vi "fgv_tim571_databuf.vi"(7 "cmd":T1, 8 "error in":errorcluster, 10 "XYZ_DATA in":cluster{"x":sgl, "y":sgl, "Z":sgl}[](array[cluster])=[{"x"=-0.23617366, "y"=0.44382635, "Z"=2.0646958e-08}, {"x"=-0.2354099, "y"=0.44731313, "Z"=2.0580186e-08}, {"x"=-0.23604421, "y"=0.44938534, "Z"=2.063564e-08}, {"x"=-0.24097842, "y"=0.44728905, "Z"=2.1067002e-08}, {"x"=-0.24088132, "y"=0.4500757, "Z"=2.1058515e-08}, {"x"=-0.2385779, "y"=0.45491207, "Z"=2.0857142e-08}, {"x"=-0.23842053, "y"=0.4576677, "Z"=2.0843386e-08}, {"x"=-0.2360333, "y"=0.46244708, "Z"=2.0634687e-08}, {"x"=-0.23433791, "y"=0.46651757, "Z"=2.0486471e-08}, {"x"=-0.24597977, "y"=0.45851648, "Z"=2.1504235e-08}, {"x"=-0.24352892, "y"=0.46327513, "Z"=2.1289974e-08}, {"x"=-0.24478552, "y"=0.46469545, "Z"=2.139983e-08}, {"x"=-0.24905264, "y"=0.46349877, "Z"=2.1772873e-08}, {"x"=-0.24651532, "y"=0.46820956, "Z"=2.1551054e-08}, {"x"=-0.2507923, "y"=0.46705818, "Z"=2.192496e-08}, {"x"=-0.24513243, "y"=0.47430584, "Z"=2.1430157e-08}, {"x"=-0.24786437, "y"=0.47445863, "Z"=2.1668992e-08}, {"x"=-0.26143128, "y"=0.46576256, "Z"=2.2855048e-08}, {"x"=-0.25101602, "y"=0.4767269, "Z"=2.1944517e-08}, {"x"=-0.26390603, "y"=0.46881858, "Z"=2.3071397e-08}, {"x"=-0.26356125, "y"=0.47159782, "Z"=2.3041256e-08}, {"x"=-0.26476908, "y"=0.47313452, "Z"=2.3146848e-08}, {"x"=-0.0015831427, "y"=0.6787779, "Z"=1.3840273e-10}, {"x"=-0.26715785, "y"=0.47622886, "Z"=2.3355682e-08}, {"x"=-0.27233183, "y"=0.47477728, "Z"=2.3808004e-08}, {"x"=-0.27913585, "y"=0.47218478, "Z"=2.4402832e-08}, {"x"=-0.27631214, "y"=0.4767745, "Z"=2.4155975e-08}, {"x"=-0.2815347, "y"=0.4754463, "Z"=2.4612545e-08}, {"x"=-0.28028262, "y"=0.47883677, "Z"=2.4503084e-08}, {"x"=-0.28144807, "y"=0.4804706, "Z"=2.4604972e-08}, {"x"=-0.28424227, "y"=0.480964, "Z"=2.4849248e-08}, {"x"=-0.29279748, "y"=0.4775015, "Z"=2.5597169e-08}, {"x"=-0.29644778, "y"=0.4775161, "Z"=2.5916288e-08}, {"x"=-0.30922702, "y"=0.4714151, "Z"=2.7033485e-08}, {"x"=-0.31209967, "y"=0.47210872, "Z"=2.7284619e-08}, {"x"=-0.30578443, "y"=0.4788735, "Z"=2.6732524e-08}, {"x"=-0.31701317, "y"=0.4741198, "Z"=2.7714172e-08}, {"x"=-0.31820545, "y"=0.4759674, "Z"=2.7818404e-08}, {"x"=-0.32023188, "y"=0.47728705, "Z"=2.799556e-08}, {"x"=-0.32564586, "y"=0.4765036, "Z"=2.8468866e-08}, {"x"=-0.33533517, "y"=0.47315145, "Z"=2.9315931e-08}, {"x"=-5.450293, "y"=-2.6383529, "Z"=4.7647976e-07}, {"x"=-5.4480753, "y"=-2.593715, "Z"=4.7628586e-07}, {"x"=-5.448104, "y"=-2.550746, "Z"=4.7628836e-07}, {"x"=-5.459038, "y"=-2.5144534, "Z"=4.772442e-07}, {"x"=-5.473198, "y"=-2.4801433, "Z"=4.7848215e-07}, {"x"=-5.4793234, "y"=-2.4413216, "Z"=4.790177e-07}, {"x"=-5.482568, "y"=-2.4010663, "Z"=4.793013e-07}, {"x"=-5.4951506, "y"=-2.3662121, "Z"=4.804013e-07}, {"x"=-5.5013714, "y"=-2.3279579, "Z"=4.809452e-07}, {"x"=-5.519656, "y"=-2.2963793, "Z"=4.8254367e-07}, {"x"=-5.533345, "y"=-2.2623425, "Z"=4.837404e-07}, {"x"=-5.53974, "y"=-2.2245321, "Z"=4.8429945e-07}, {"x"=-5.5441055, "y"=-2.1858287, "Z"=4.846811e-07}, {"x"=-5.5499907, "y"=-2.148081, "Z"=4.851956e-07}, {"x"=-5.5520506, "y"=-2.108567, "Z"=4.8537566e-07}, {"x"=-5.572659, "y"=-2.0784407, "Z"=4.871773e-07}, {"x"=-5.580522, "y"=-2.0420315, "Z"=4.878647e-07}, {"x"=-5.593558, "y"=-2.008223, "Z"=4.890044e-07}, {"x"=-5.610909, "y"=-1.976495, "Z"=4.9052124e-07}, {"x"=-5.6398616, "y"=-1.9501503, "Z"=4.9305237e-07}, {"x"=-5.665971, "y"=-1.9223063, "Z"=4.953349e-07}, {"x"=-5.6819243, "y"=-1.8897145, "Z"=4.967296e-07}, {"x"=-5.683987, "y"=-1.8509235, "Z"=4.9690993e-07}, {"x"=-5.6995296, "y"=-1.8182178, "Z"=4.982687e-07}, {"x"=-5.7130475, "y"=-1.7846243, "Z"=4.994505e-07}, {"x"=-5.740175, "y"=-1.7568197, "Z"=5.01822e-07}, {"x"=-5.7644033, "y"=-1.7276263, "Z"=5.0394016e-07}, {"x"=-5.7727613, "y"=-1.6917732, "Z"=5.046708e-07}, {"x"=-5.77997, "y"=-1.6555295, "Z"=5.0530105e-07}, {"x"=-5.814833, "y"=-1.6303596, "Z"=5.083489e-07}, {"x"=-5.842147, "y"=-1.6019523, "Z"=5.107367e-07}, {"x"=-5.868392, "y"=-1.5729468, "Z"=5.130311e-07}, {"x"=-5.886077, "y"=-1.5405362, "Z"=5.145772e-07}, {"x"=-5.8923306, "y"=-1.5038257, "Z"=5.1512393e-07}, {"x"=-5.9086933, "y"=-1.4708805, "Z"=5.165544e-07}, {"x"=-5.9060388, "y"=-1.4310868, "Z"=5.163223e-07}, {"x"=-5.9021783, "y"=-1.3910661, "Z"=5.159848e-07}, {"x"=-5.8857613, "y"=-1.3469288, "Z"=5.145496e-07}, {"x"=-5.8766103, "y"=-1.305614, "Z"=5.1374957e-07}, {"x"=-5.8567367, "y"=-1.2610137, "Z"=5.120122e-07}, {"x"=-5.8346424, "y"=-1.2160943, "Z"=5.1008067e-07}, {"x"=-5.8446207, "y"=-1.1818175, "Z"=5.10953e-07}, {"x"=-5.8887625, "y"=-1.1582162, "Z"=5.14812e-07}, {"x"=-5.9538646, "y"=-1.1405971, "Z"=5.2050336e-07}, {"x"=-5.9461527, "y"=-1.1004817, "Z"=5.198292e-07}, {"x"=-5.934338, "y"=-1.0593927, "Z"=5.187963e-07}, {"x"=-5.9155188, "y"=-1.0165718, "Z"=5.171511e-07}, {"x"=-5.947433, "y"=-0.98834354, "Z"=5.199411e-07}, {"x"=-6.0419035, "y"=-0.9769929, "Z"=5.2819996e-07}, {"x"=-6.122918, "y"=-0.9609745, "Z"=5.352825e-07}, {"x"=-6.0530334, "y"=-0.90456265, "Z"=5.29173e-07}, {"x"=-5.893567, "y"=-0.8262395, "Z"=5.15232e-07}, {"x"=-5.918724, "y"=-0.7960438, "Z"=5.174313e-07}, {"x"=-5.8494763, "y"=-0.74268264, "Z"=5.1137744e-07}, {"x"=-5.8722486, "y"=-0.7120914, "Z"=5.1336826e-07}, {"x"=-5.9046063, "y"=-0.68353313, "Z"=5.161971e-07}, {"x"=-5.9124384, "y"=-0.6491621, "Z"=5.1688176e-07}, {"x"=-5.9542623, "y"=-0.62222403, "Z"=5.2053815e-07}, {"x"=-5.9969497, "y"=-0.59505194, "Z"=5.2427e-07}, {"x"=-5.9670506, "y"=-0.5524588, "Z"=5.2165615e-07}, {"x"=-5.984905, "y"=-0.51988906, "Z"=5.23217e-07}, {"x"=-6.0271215, "y"=-0.49192494, "Z"=5.269077e-07}, {"x"=-6.070197, "y"=-0.4636951, "Z"=5.306735e-07}, {"x"=-6.0796986, "y"=-0.4289028, "Z"=5.3150416e-07}, {"x"=-6.024004, "y"=-0.3825739, "Z"=5.266352e-07}, {"x"=-5.968964, "y"=-0.33709878, "Z"=5.2182344e-07}, {"x"=-5.966886, "y"=-0.30106133, "Z"=5.2164177e-07}, {"x"=-5.954714, "y"=-0.26351756, "Z"=5.205776e-07}, {"x"=-5.9442844, "y"=-0.22645015, "Z"=5.1966583e-07}, {"x"=-5.9830976, "y"=-0.19678587, "Z"=5.23059e-07}, {"x"=-5.978194, "y"=-0.16057408, "Z"=5.2263033e-07}, {"x"=-5.967126, "y"=-0.123648226, "Z"=5.2166274e-07}, {"x"=-5.9211173, "y"=-0.08240992, "Z"=5.176405e-07}, {"x"=-5.8559747, "y"=-0.039417505, "Z"=5.119456e-07}, {"x"=-5.871979, "y"=-0.0067341924, "Z"=5.1334473e-07}, {"x"=-5.889789, "y"=0.02589035, "Z"=5.149017e-07}, {"x"=-5.8646536, "y"=0.06319648, "Z"=5.127043e-07}, {"x"=-5.8402796, "y"=0.10008913, "Z"=5.1057344e-07}, {"x"=-5.825632, "y"=0.13574708, "Z"=5.0929293e-07}, {"x"=-5.8336806, "y"=0.1692087, "Z"=5.0999654e-07}, {"x"=-5.824593, "y"=0.20412987, "Z"=5.092021e-07}, {"x"=-5.839228, "y"=0.23711291, "Z"=5.104815e-07}, {"x"=-5.8626547, "y"=0.2696217, "Z"=5.1252954e-07}, {"x"=-5.959748, "y"=0.2976503, "Z"=5.210177e-07}, {"x"=-5.9758472, "y"=0.33151048, "Z"=5.224252e-07}, {"x"=-5.952808, "y"=0.367589, "Z"=5.20411e-07}, {"x"=-5.9215603, "y"=0.40376043, "Z"=5.1767927e-07}, {"x"=-5.947047, "y"=0.4372328, "Z"=5.1990736e-07}, {"x"=-5.9403634, "y"=0.47211158, "Z"=5.1932307e-07}, {"x"=-5.9364743, "y"=0.50681686, "Z"=5.189831e-07}, {"x"=-5.9393806, "y"=0.5413065, "Z"=5.192371e-07}, {"x"=-5.9390874, "y"=0.5758766, "Z"=5.192115e-07}, {"x"=-5.930593, "y"=0.61053234, "Z"=5.184689e-07}, {"x"=-5.921897, "y"=0.64508575, "Z"=5.1770866e-07}, {"x"=-5.8849998, "y"=0.6795378, "Z"=5.14483e-07}, {"x"=-5.8789034, "y"=0.7137373, "Z"=5.1395006e-07}, {"x"=-5.881607, "y"=0.74796987, "Z"=5.141864e-07}, {"x"=-5.901109, "y"=0.7825303, "Z"=5.158914e-07}, {"x"=-5.934404, "y"=0.81764466, "Z"=5.1880204e-07}, {"x"=-5.96449, "y"=0.85306275, "Z"=5.214323e-07}, {"x"=-6.003358, "y"=0.88914883, "Z"=5.248302e-07}, {"x"=-6.011032, "y"=0.9244334, "Z"=5.255011e-07}, {"x"=-5.98953, "y"=0.9584675, "Z"=5.2362134e-07}, {"x"=-5.948862, "y"=0.99126697, "Z"=5.2006607e-07}, {"x"=-5.946951, "y"=1.0258671, "Z"=5.1989895e-07}, {"x"=-5.9398484, "y"=1.0601362, "Z"=5.1927805e-07}, {"x"=-5.9375367, "y"=1.0946827, "Z"=5.1907597e-07}, {"x"=-5.9370184, "y"=1.1293662, "Z"=5.190306e-07}, {"x"=-5.924337, "y"=1.1630824, "Z"=5.17922e-07}, {"x"=-5.919434, "y"=1.1973629, "Z"=5.174934e-07}, {"x"=-5.8755016, "y"=1.227981, "Z"=5.1365265e-07}, {"x"=-5.8821654, "y"=1.2631369, "Z"=5.1423524e-07}, {"x"=-5.8836465, "y"=1.2978667, "Z"=5.1436473e-07}, {"x"=-5.877965, "y"=1.3318619, "Z"=5.1386803e-07}, {"x"=-5.872087, "y"=1.3658118, "Z"=5.1335417e-07}, {"x"=-5.8967824, "y"=1.4034905, "Z"=5.155131e-07}, {"x"=-5.9073515, "y"=1.4396942, "Z"=5.1643707e-07}, {"x"=-5.930582, "y"=1.4777781, "Z"=5.1846797e-07}, {"x"=-5.932773, "y"=1.5132372, "Z"=5.186595e-07}, {"x"=-5.9208994, "y"=1.5467211, "Z"=5.1762146e-07}, {"x"=-5.90686, "y"=1.5797939, "Z"=5.163941e-07}, {"x"=-5.9114027, "y"=1.6157031, "Z"=5.1679126e-07}, {"x"=-5.921648, "y"=1.6526682, "Z"=5.176869e-07}, {"x"=-5.952365, "y"=1.6933084, "Z"=5.203723e-07}, {"x"=-5.9562182, "y"=1.7296524, "Z"=5.2070914e-07}, {"x"=-5.960833, "y"=1.7662549, "Z"=5.2111255e-07}, {"x"=-5.955396, "y"=1.8010967, "Z"=5.206373e-07}, {"x"=-5.9360123, "y"=1.8332419, "Z"=5.1894267e-07}, {"x"=-5.9546967, "y"=1.87286, "Z"=5.205761e-07}, {"x"=-5.9525537, "y"=1.9084897, "Z"=5.2038877e-07}, {"x"=-5.962914, "y"=1.9468365, "Z"=5.212945e-07}, {"x"=-5.9730287, "y"=1.9853451, "Z"=5.2217877e-07}, {"x"=-5.9907017, "y"=2.0257678, "Z"=5.2372377e-07}, {"x"=-6.012978, "y"=2.0675642, "Z"=5.256712e-07}, {"x"=-6.018428, "y"=2.1057465, "Z"=5.261477e-07}, {"x"=-5.995456, "y"=2.1371899, "Z"=5.241394e-07}, {"x"=-5.9985223, "y"=2.1749434, "Z"=5.244075e-07}, {"x"=-5.949031, "y"=2.199419, "Z"=5.200808e-07}, {"x"=-5.8984914, "y"=2.2231166, "Z"=5.156625e-07}, {"x"=-5.8836193, "y"=2.2558508, "Z"=5.1436234e-07}, {"x"=-5.9023213, "y"=2.2977157, "Z"=5.159973e-07}, {"x"=-5.9255486, "y"=2.3412008, "Z"=5.180279e-07}, {"x"=-5.926359, "y"=2.3786733, "Z"=5.180988e-07}, {"x"=-5.9173374, "y"=2.4134002, "Z"=5.1731007e-07}, {"x"=-5.9282303, "y"=2.4541004, "Z"=5.1826237e-07}, {"x"=-5.9598885, "y"=2.5014155, "Z"=5.2103e-07}, {"x"=-5.97974, "y"=2.5455847, "Z"=5.227655e-07}, {"x"=-5.9897494, "y"=2.5870125, "Z"=5.2364055e-07}, {"x"=-5.9861636, "y"=2.6242948, "Z"=5.2332706e-07}, {"x"=-6.0307593, "y"=2.6776361, "Z"=5.272257e-07}, {"x"=-6.0275636, "y"=2.715564, "Z"=5.2694634e-07}, {"x"=-6.012784, "y"=2.7496164, "Z"=5.256543e-07}, {"x"=-6.020459, "y"=2.7915087, "Z"=5.2632527e-07}, {"x"=-6.0335007, "y"=2.8355787, "Z"=5.274654e-07}, {"x"=-6.0199194, "y"=2.8702981, "Z"=5.262781e-07}, {"x"=-6.032395, "y"=2.914659, "Z"=5.273687e-07}, {"x"=-6.0249076, "y"=2.9518294, "Z"=5.2671413e-07}, {"x"=-6.0424, "y"=2.9986615, "Z"=5.282434e-07}, {"x"=-6.0418506, "y"=3.0388634, "Z"=5.2819536e-07}, {"x"=-6.0772843, "y"=3.0935318, "Z"=5.312931e-07}, {"x"=-6.1122847, "y"=3.148692, "Z"=5.343529e-07}, {"x"=-6.07932, "y"=3.1766086, "Z"=5.31471e-07}, {"x"=-6.0849957, "y"=3.2204063, "Z"=5.319672e-07}, {"x"=-6.1096983, "y"=3.2725575, "Z"=5.341268e-07}, {"x"=-6.1174703, "y"=3.3179538, "Z"=5.3480625e-07}, {"x"=-6.0983577, "y"=3.3518903, "Z"=5.3313533e-07}, {"x"=-6.0909343, "y"=3.3909798, "Z"=5.324864e-07}, {"x"=-6.100575, "y"=3.4378998, "Z"=5.333292e-07}, {"x"=-6.1198716, "y"=3.489613, "Z"=5.3501617e-07}, {"x"=-6.1170197, "y"=3.5315034, "Z"=5.3476685e-07}, {"x"=-6.096713, "y"=3.5653276, "Z"=5.329916e-07}, {"x"=-6.0960503, "y"=3.6085389, "Z"=5.3293365e-07}, {"x"=-6.0959897, "y"=3.6522777, "Z"=5.3292837e-07}, {"x"=-6.125203, "y"=3.7107499, "Z"=5.354823e-07}, {"x"=-6.119087, "y"=3.7521627, "Z"=5.349476e-07}, {"x"=-6.0886374, "y"=3.781352, "Z"=5.322856e-07}, {"x"=-6.0811543, "y"=3.8222268, "Z"=5.316314e-07}, {"x"=-6.073401, "y"=3.8631191, "Z"=5.3095357e-07}, {"x"=-6.090102, "y"=3.9171696, "Z"=5.3241365e-07}, {"x"=-6.116061, "y"=3.9767406, "Z"=5.3468307e-07}, {"x"=-6.139777, "y"=4.0357633, "Z"=5.367564e-07}, {"x"=-6.2014976, "y"=4.1164994, "Z"=5.421521e-07}, {"x"=-6.416801, "y"=4.2847557, "Z"=5.6097457e-07}, {"x"=-6.5773406, "y"=4.4254436, "Z"=5.750094e-07}, {"x"=-6.599612, "y"=4.489136, "Z"=5.7695644e-07}, {"x"=-6.5730267, "y"=4.524938, "Z"=5.746322e-07}, {"x"=-6.536785, "y"=4.55495, "Z"=5.714639e-07}, {"x"=-6.5372787, "y"=4.6068134, "Z"=5.7150703e-07}, {"x"=-6.4963865, "y"=4.6338573, "Z"=5.6793215e-07}, {"x"=-6.481788, "y"=4.6768293, "Z"=5.666559e-07}, {"x"=-6.3888826, "y"=4.6710234, "Z"=5.585339e-07}, {"x"=-6.3376727, "y"=4.6904745, "Z"=5.5405695e-07}, {"x"=-6.31171, "y"=4.725655, "Z"=5.517872e-07}, {"x"=-6.238583, "y"=4.7301755, "Z"=5.4539424e-07}, {"x"=-6.1814947, "y"=4.744422, "Z"=5.4040345e-07}, {"x"=-6.142764, "y"=4.7703357, "Z"=5.370175e-07}, {"x"=-6.0981383, "y"=4.7920227, "Z"=5.331162e-07}, {"x"=-6.073289, "y"=4.8268633, "Z"=5.309438e-07}, {"x"=-0.0016451083, "y"=0.6811374, "Z"=1.4381994e-10}, {"x"=-6.4596453, "y"=5.2017484, "Z"=5.6472015e-07}, {"x"=-6.502582, "y"=5.288397, "Z"=5.6847375e-07}, {"x"=-6.4837894, "y"=5.331975, "Z"=5.6683086e-07}, {"x"=-6.493028, "y"=5.3960586, "Z"=5.6763855e-07}, {"x"=0.0, "y"=0.68, "Z"=0.0}, {"x"=-7.0161138, "y"=5.9017487, "Z"=6.133682e-07}, {"x"=-6.989613, "y"=5.9454827, "Z"=6.110514e-07}, {"x"=-7.0041914, "y"=6.0206146, "Z"=6.1232583e-07}, {"x"=-6.998339, "y"=6.080819, "Z"=6.1181424e-07}, {"x"=-6.9975395, "y"=6.1454444, "Z"=6.117443e-07}, {"x"=-7.0276036, "y"=6.2350473, "Z"=6.143726e-07}, {"x"=-7.1029325, "y"=6.362039, "Z"=6.209581e-07}, {"x"=-7.2088842, "y"=6.5158896, "Z"=6.3022065e-07}, {"x"=-7.1601167, "y"=6.5456853, "Z"=6.259573e-07}, {"x"=-7.1512794, "y"=6.6082983, "Z"=6.251847e-07}, {"x"=-7.1205034, "y"=6.653012, "Z"=6.2249416e-07}, {"x"=-7.086399, "y"=6.6949787, "Z"=6.1951266e-07}, {"x"=-7.048255, "y"=6.7334933, "Z"=6.16178e-07}, {"x"=-7.0808544, "y"=6.833427, "Z"=6.1902796e-07}, {"x"=-7.048694, "y"=6.877815, "Z"=6.162164e-07}, {"x"=-7.003556, "y"=6.910737, "Z"=6.122703e-07}, {"x"=-7.0861115, "y"=7.058415, "Z"=6.1948754e-07}, {"x"=-7.1871443, "y"=7.225441, "Z"=6.283201e-07}, {"x"=-7.2004256, "y"=7.3145723, "Z"=6.294812e-07}, {"x"=-7.218032, "y"=7.408851, "Z"=6.310204e-07}, {"x"=-7.145303, "y"=7.4191637, "Z"=6.246622e-07}, {"x"=-7.019162, "y"=7.377773, "Z"=6.1363465e-07}, {"x"=-6.992312, "y"=7.4302983, "Z"=6.112873e-07}, {"x"=-6.945772, "y"=7.4638724, "Z"=6.072187e-07}, {"x"=-6.8535547, "y"=7.45215, "Z"=5.991568e-07}, {"x"=-6.8373823, "y"=7.5152345, "Z"=5.9774294e-07}, {"x"=-6.828441, "y"=7.586181, "Z"=5.969613e-07}, {"x"=-6.711966, "y"=7.547832, "Z"=5.867787e-07}, {"x"=-6.6600904, "y"=7.5745335, "Z"=5.822436e-07}, {"x"=-6.76213, "y"=7.762151, "Z"=5.9116417e-07}, {"x"=-6.7496448, "y"=7.8319125, "Z"=5.9007266e-07}, {"x"=0.0, "y"=0.68, "Z"=0.0}, {"x"=0.0, "y"=0.68, "Z"=0.0}, {"x"=0.0, "y"=0.68, "Z"=0.0}, {"x"=0.0, "y"=0.68, "Z"=0.0}, {"x"=0.0, "y"=0.68, "Z"=0.0}, {"x"=0.0, "y"=0.68, "Z"=0.0}, {"x"=0.0, "y"=0.68, "Z"=0.0}, {"x"=0.0, "y"=0.68, "Z"=0.0}, {"x"=0.0, "y"=0.68, "Z"=0.0}, {"x"=0.0, "y"=0.68, "Z"=0.0}, {"x"=-6.6047463, "y"=8.642182, "Z"=5.774053e-07}, {"x"=-6.5773363, "y"=8.70367, "Z"=5.75009e-07}, {"x"=-6.549433, "y"=8.765107, "Z"=5.7256966e-07}, {"x"=0.0, "y"=0.68, "Z"=0.0}, {"x"=0.0, "y"=0.68, "Z"=0.0}, {"x"=0.0, "y"=0.68, "Z"=0.0}, {"x"=0.0, "y"=0.68, "Z"=0.0}, {"x"=0.0, "y"=0.68, "Z"=0.0}, {"x"=0.0, "y"=0.68, "Z"=0.0}, {"x"=0.0, "y"=0.68, "Z"=0.0}, {"x"=0.0, "y"=0.68, "Z"=0.0}, {"x"=0.0, "y"=0.68, "Z"=0.0}, {"x"=0.0, "y"=0.68, "Z"=0.0}, {"x"=0.0, "y"=0.68, "Z"=0.0}, {"x"=0.0, "y"=0.68, "Z"=0.0}, {"x"=0.0, "y"=0.68, "Z"=0.0}, {"x"=-6.206232, "y"=9.763209, "Z"=5.4256606e-07}, {"x"=0.0, "y"=0.68, "Z"=0.0}, {"x"=0.0, "y"=0.68, "Z"=0.0}, {"x"=0.0, "y"=0.68, "Z"=0.0}, {"x"=0.0, "y"=0.68, "Z"=0.0}, {"x"=0.0, "y"=0.68, "Z"=0.0}, {"x"=0.0, "y"=0.68, "Z"=0.0}, {"x"=0.0, "y"=0.68, "Z"=0.0}, {"x"=0.0, "y"=0.68, "Z"=0.0}, {"x"=0.0, "y"=0.68, "Z"=0.0}, {"x"=0.0, "y"=0.68, "Z"=0.0}, {"x"=0.0, "y"=0.68, "Z"=0.0}, {"x"=0.0, "y"=0.68, "Z"=0.0}, {"x"=0.0, "y"=0.68, "Z"=0.0}, {"x"=0.0, "y"=0.68, "Z"=0.0}, {"x"=0.0, "y"=0.68, "Z"=0.0}, {"x"=0.0, "y"=0.68, "Z"=0.0}, {"x"=0.0, "y"=0.68, "Z"=0.0}, {"x"=0.0, "y"=0.68, "Z"=0.0}, {"x"=0.0, "y"=0.68, "Z"=0.0}, {"x"=0.0, "y"=0.68, "Z"=0.0}, {"x"=0.0, "y"=0.68, "Z"=0.0}, {"x"=0.0, "y"=0.68, "Z"=0.0}, {"x"=0.0, "y"=0.68, "Z"=0.0}, {"x"=0.0, "y"=0.68, "Z"=0.0}, {"x"=0.0, "y"=0.68, "Z"=0.0}, {"x"=0.0, "y"=0.68, "Z"=0.0}, {"x"=0.0, "y"=0.68, "Z"=0.0}, {"x"=0.0, "y"=0.68, "Z"=0.0}, {"x"=0.0, "y"=0.68, "Z"=0.0}, {"x"=0.0, "y"=0.68, "Z"=0.0}, {"x"=0.0, "y"=0.68, "Z"=0.0}, {"x"=0.0, "y"=0.68, "Z"=0.0}, {"x"=0.0, "y"=0.68, "Z"=0.0}, {"x"=0.0, "y"=0.68, "Z"=0.0}, {"x"=0.0, "y"=0.68, "Z"=0.0}, {"x"=0.0, "y"=0.68, "Z"=0.0}, {"x"=0.0, "y"=0.68, "Z"=0.0}, {"x"=0.0, "y"=0.68, "Z"=0.0}, {"x"=0.0, "y"=0.68, "Z"=0.0}, {"x"=0.0, "y"=0.68, "Z"=0.0}, {"x"=0.0, "y"=0.68, "Z"=0.0}, {"x"=0.0, "y"=0.68, "Z"=0.0}, {"x"=0.0, "y"=0.68, "Z"=0.0}, {"x"=0.0, "y"=0.68, "Z"=0.0}, {"x"=0.0, "y"=0.68, "Z"=0.0}, {"x"=0.0, "y"=0.68, "Z"=0.0}, {"x"=0.0, "y"=0.68, "Z"=0.0}, {"x"=0.0, "y"=0.68, "Z"=0.0}, {"x"=0.0, "y"=0.68, "Z"=0.0}, {"x"=0.0, "y"=0.68, "Z"=0.0}, {"x"=0.0, "y"=0.68, "Z"=0.0}, {"x"=0.0, "y"=0.68, "Z"=0.0}, {"x"=0.0, "y"=0.68, "Z"=0.0}, {"x"=0.0, "y"=0.68, "Z"=0.0}, {"x"=0.0, "y"=0.68, "Z"=0.0}, {"x"=0.0, "y"=0.68, "Z"=0.0}, {"x"=0.0, "y"=0.68, "Z"=0.0}, {"x"=0.0, "y"=0.68, "Z"=0.0}, {"x"=0.0, "y"=0.68, "Z"=0.0}, {"x"=0.0, "y"=0.68, "Z"=0.0}, {"x"=0.0, "y"=0.68, "Z"=0.0}, {"x"=0.0, "y"=0.68, "Z"=0.0}, {"x"=0.0, "y"=0.68, "Z"=0.0}, {"x"=0.0, "y"=0.68, "Z"=0.0}, {"x"=0.0, "y"=0.68, "Z"=0.0}, {"x"=0.0, "y"=0.68, "Z"=0.0}, {"x"=0.0, "y"=0.68, "Z"=0.0}, {"x"=0.0, "y"=0.68, "Z"=0.0}, {"x"=0.0, "y"=0.68, "Z"=0.0}, {"x"=0.0, "y"=0.68, "Z"=0.0}, {"x"=0.0, "y"=0.68, "Z"=0.0}, {"x"=0.0, "y"=0.68, "Z"=0.0}, {"x"=0.0, "y"=0.68, "Z"=0.0}, {"x"=0.0, "y"=0.68, "Z"=0.0}, {"x"=0.0, "y"=0.68, "Z"=0.0}, {"x"=0.0, "y"=0.68, "Z"=0.0}, {"x"=0.0, "y"=0.68, "Z"=0.0}, {"x"=0.0, "y"=0.68, "Z"=0.0}, {"x"=0.0, "y"=0.68, "Z"=0.0}, {"x"=0.0, "y"=0.68, "Z"=0.0}, {"x"=0.0, "y"=0.68, "Z"=0.0}, {"x"=0.0, "y"=0.68, "Z"=0.0}, {"x"=0.0, "y"=0.68, "Z"=0.0}, {"x"=0.0, "y"=0.68, "Z"=0.0}, {"x"=0.0, "y"=0.68, "Z"=0.0}, {"x"=0.0, "y"=0.68, "Z"=0.0}, {"x"=0.0, "y"=0.68, "Z"=0.0}, {"x"=0.0, "y"=0.68, "Z"=0.0}, {"x"=0.0, "y"=0.68, "Z"=0.0}, {"x"=0.0, "y"=0.68, "Z"=0.0}, {"x"=0.0, "y"=0.68, "Z"=0.0}, {"x"=0.0, "y"=0.68, "Z"=0.0}, {"x"=0.0, "y"=0.68, "Z"=0.0}, {"x"=0.0, "y"=0.68, "Z"=0.0}, {"x"=0.0, "y"=0.68, "Z"=0.0}, {"x"=0.0, "y"=0.68, "Z"=0.0}, {"x"=0.0, "y"=0.68, "Z"=0.0}, {"x"=0.0, "y"=0.68, "Z"=0.0}, {"x"=0.0, "y"=0.68, "Z"=0.0}, {"x"=0.0, "y"=0.68, "Z"=0.0}, {"x"=0.0, "y"=0.68, "Z"=0.0}, {"x"=0.0, "y"=0.68, "Z"=0.0}, {"x"=0.0, "y"=0.68, "Z"=0.0}, {"x"=0.0, "y"=0.68, "Z"=0.0}, {"x"=0.0, "y"=0.68, "Z"=0.0}, {"x"=0.0, "y"=0.68, "Z"=0.0}, {"x"=0.0, "y"=0.68, "Z"=0.0}, {"x"=0.0, "y"=0.68, "Z"=0.0}, {"x"=0.0, "y"=0.68, "Z"=0.0}, {"x"=0.0, "y"=0.68, "Z"=0.0}, {"x"=0.0, "y"=0.68, "Z"=0.0}, {"x"=0.0, "y"=0.68, "Z"=0.0}, {"x"=0.0, "y"=0.68, "Z"=0.0}, {"x"=0.0, "y"=0.68, "Z"=0.0}, {"x"=0.0, "y"=0.68, "Z"=0.0}, {"x"=0.0, "y"=0.68, "Z"=0.0}, {"x"=0.0, "y"=0.68, "Z"=0.0}, {"x"=0.0, "y"=0.68, "Z"=0.0}, {"x"=0.0, "y"=0.68, "Z"=0.0}, {"x"=0.0, "y"=0.68, "Z"=0.0}, {"x"=0.0, "y"=0.68, "Z"=0.0}, {"x"=0.0, "y"=0.68, "Z"=0.0}, {"x"=0.0, "y"=0.68, "Z"=0.0}, {"x"=0.0, "y"=0.68, "Z"=0.0}, {"x"=0.0, "y"=0.68, "Z"=0.0}, {"x"=0.0, "y"=0.68, "Z"=0.0}, {"x"=0.0, "y"=0.68, "Z"=0.0}, {"x"=0.0, "y"=0.68, "Z"=0.0}, {"x"=0.0, "y"=0.68, "Z"=0.0}, {"x"=0.0, "y"=0.68, "Z"=0.0}, {"x"=0.0, "y"=0.68, "Z"=0.0}, {"x"=0.0, "y"=0.68, "Z"=0.0}, {"x"=0.0, "y"=0.68, "Z"=0.0}, {"x"=0.0, "y"=0.68, "Z"=0.0}, {"x"=0.0, "y"=0.68, "Z"=0.0}, {"x"=0.0, "y"=0.68, "Z"=0.0}, {"x"=0.0, "y"=0.68, "Z"=0.0}, {"x"=0.0, "y"=0.68, "Z"=0.0}, {"x"=0.0, "y"=0.68, "Z"=0.0}, {"x"=0.0, "y"=0.68, "Z"=0.0}, {"x"=0.0, "y"=0.68, "Z"=0.0}, {"x"=0.0, "y"=0.68, "Z"=0.0}, {"x"=0.0, "y"=0.68, "Z"=0.0}, {"x"=0.0, "y"=0.68, "Z"=0.0}, {"x"=0.0, "y"=0.68, "Z"=0.0}, {"x"=0.0, "y"=0.68, "Z"=0.0}, {"x"=0.0, "y"=0.68, "Z"=0.0}, {"x"=0.0, "y"=0.68, "Z"=0.0}, {"x"=0.0, "y"=0.68, "Z"=0.0}, {"x"=0.0, "y"=0.68, "Z"=0.0}, {"x"=0.0, "y"=0.68, "Z"=0.0}, {"x"=0.0, "y"=0.68, "Z"=0.0}, {"x"=0.0, "y"=0.68, "Z"=0.0}, {"x"=0.0, "y"=0.68, "Z"=0.0}, {"x"=0.0, "y"=0.68, "Z"=0.0}, {"x"=0.0, "y"=0.68, "Z"=0.0}, {"x"=0.0, "y"=0.68, "Z"=0.0}, {"x"=0.0, "y"=0.68, "Z"=0.0}, {"x"=0.0, "y"=0.68, "Z"=0.0}, {"x"=0.0, "y"=0.68, "Z"=0.0}, {"x"=0.0, "y"=0.68, "Z"=0.0}, {"x"=0.0, "y"=0.68, "Z"=0.0}, {"x"=0.0, "y"=0.68, "Z"=0.0}, {"x"=0.0, "y"=0.68, "Z"=0.0}, {"x"=0.0, "y"=0.68, "Z"=0.0}, {"x"=0.0, "y"=0.68, "Z"=0.0}, {"x"=0.0, "y"=0.68, "Z"=0.0}, {"x"=0.0, "y"=0.68, "Z"=0.0}, {"x"=0.0, "y"=0.68, "Z"=0.0}, {"x"=0.0, "y"=0.68, "Z"=0.0}, {"x"=0.0, "y"=0.68, "Z"=0.0}, {"x"=0.0, "y"=0.68, "Z"=0.0}, {"x"=0.0, "y"=0.68, "Z"=0.0}, {"x"=0.0, "y"=0.68, "Z"=0.0}, {"x"=0.0, "y"=0.68, "Z"=0.0}, {"x"=0.0, "y"=0.68, "Z"=0.0}, {"x"=0.0, "y"=0.68, "Z"=0.0}, {"x"=0.0, "y"=0.68, "Z"=0.0}, {"x"=0.0, "y"=0.68, "Z"=0.0}, {"x"=0.0, "y"=0.68, "Z"=0.0}, {"x"=0.0, "y"=0.68, "Z"=0.0}, {"x"=0.0, "y"=0.68, "Z"=0.0}, {"x"=0.0, "y"=0.68, "Z"=0.0}, {"x"=0.0, "y"=0.68, "Z"=0.0}, {"x"=0.0, "y"=0.68, "Z"=0.0}, {"x"=0.0, "y"=0.68, "Z"=0.0}, {"x"=0.0, "y"=0.68, "Z"=0.0}, {"x"=0.0, "y"=0.68, "Z"=0.0}, {"x"=0.0, "y"=0.68, "Z"=0.0}, {"x"=0.0, "y"=0.68, "Z"=0.0}, {"x"=0.0, "y"=0.68, "Z"=0.0}, {"x"=0.0, "y"=0.68, "Z"=0.0}, {"x"=0.0, "y"=0.68, "Z"=0.0}, {"x"=0.0, "y"=0.68, "Z"=0.0}, {"x"=0.0, "y"=0.68, "Z"=0.0}, {"x"=0.0, "y"=0.68, "Z"=0.0}, {"x"=0.0, "y"=0.68, "Z"=0.0}, {"x"=5.316029, "y"=9.30421, "Z"=-4.6474202e-07}, {"x"=5.351277, "y"=9.249391, "Z"=-4.6782347e-07}, {"x"=5.3833942, "y"=9.1902275, "Z"=-4.7063128e-07}, {"x"=0.0, "y"=0.68, "Z"=0.0}, {"x"=0.0, "y"=0.68, "Z"=0.0}, {"x"=0.0, "y"=0.68, "Z"=0.0}, {"x"=5.9229383, "y"=9.5779505, "Z"=-5.177997e-07}, {"x"=6.0003104, "y"=9.581489, "Z"=-5.245638e-07}, {"x"=6.0999103, "y"=9.616638, "Z"=-5.332711e-07}, {"x"=6.13701, "y"=9.559614, "Z"=-5.3651445e-07}, {"x"=6.04924, "y"=9.324669, "Z"=-5.288414e-07}, {"x"=5.994213, "y"=9.140826, "Z"=-5.240307e-07}, {"x"=6.1913676, "y"=9.312213, "Z"=-5.4126656e-07}, {"x"=6.417741, "y"=9.518808, "Z"=-5.610567e-07}, {"x"=6.4666796, "y"=9.478103, "Z"=-5.653351e-07}, {"x"=0.0, "y"=0.68, "Z"=0.0}, {"x"=5.907469, "y"=8.524375, "Z"=-5.164473e-07}, {"x"=5.778412, "y"=8.26083, "Z"=-5.051648e-07}, {"x"=5.659322, "y"=8.015687, "Z"=-4.9475364e-07}, {"x"=5.704976, "y"=7.9865823, "Z"=-4.9874484e-07}, {"x"=5.8186827, "y"=8.043502, "Z"=-5.086854e-07}, {"x"=5.830191, "y"=7.9704795, "Z"=-5.096915e-07}, {"x"=5.8221755, "y"=7.874254, "Z"=-5.0899075e-07}, {"x"=5.875332, "y"=7.85419, "Z"=-5.136378e-07}, {"x"=5.902928, "y"=7.802952, "Z"=-5.1605036e-07}, {"x"=6.019442, "y"=7.858143, "Z"=-5.2623636e-07}, {"x"=6.089565, "y"=7.856555, "Z"=-5.3236664e-07}, {"x"=6.180717, "y"=7.878672, "Z"=-5.4033546e-07}, {"x"=6.277578, "y"=7.9060087, "Z"=-5.488033e-07}, {"x"=6.357798, "y"=7.9129314, "Z"=-5.5581637e-07}, {"x"=6.4901466, "y"=7.977448, "Z"=-5.673866e-07}, {"x"=6.529143, "y"=7.935854, "Z"=-5.707958e-07}, {"x"=6.6789546, "y"=8.016062, "Z"=-5.8389276e-07}, {"x"=6.8692126, "y"=8.137428, "Z"=-6.0052565e-07}, {"x"=7.0672393, "y"=8.263409, "Z"=-6.1783766e-07}, {"x"=7.177091, "y"=8.292017, "Z"=-6.2744124e-07}, {"x"=0.0, "y"=0.68, "Z"=0.0}, {"x"=7.342941, "y"=8.288593, "Z"=-6.419403e-07}, {"x"=7.3556395, "y"=8.213552, "Z"=-6.4305044e-07}, {"x"=7.387392, "y"=8.158542, "Z"=-6.4582633e-07}, {"x"=7.4032025, "y"=8.087855, "Z"=-6.4720854e-07}, {"x"=7.436927, "y"=8.035523, "Z"=-6.501568e-07}, {"x"=0.0, "y"=0.68, "Z"=0.0}, {"x"=0.0, "y"=0.68, "Z"=0.0}, {"x"=0.0, "y"=0.68, "Z"=0.0}, {"x"=0.0, "y"=0.68, "Z"=0.0}, {"x"=6.662852, "y"=6.8971677, "Z"=-5.8248503e-07}, {"x"=6.7562423, "y"=6.911185, "Z"=-5.9064945e-07}, {"x"=0.0014780493, "y"=0.68134737, "Z"=-1.2921518e-10}, {"x"=6.9263463, "y"=6.920517, "Z"=-6.055204e-07}, {"x"=7.0080867, "y"=6.920687, "Z"=-6.126664e-07}, {"x"=5.7576256, "y"=5.74741, "Z"=-5.033476e-07}, {"x"=5.7296643, "y"=5.6639524, "Z"=-5.009032e-07}, {"x"=6.963505, "y"=6.666409, "Z"=-6.087689e-07}, {"x"=6.947913, "y"=6.583066, "Z"=-6.0740587e-07}, {"x"=6.831265, "y"=6.415871, "Z"=-5.9720816e-07}, {"x"=6.7529287, "y"=6.2834435, "Z"=-5.903598e-07}, {"x"=6.694938, "y"=6.169878, "Z"=-5.852901e-07}, {"x"=6.7267604, "y"=6.13084, "Z"=-5.8807206e-07}, {"x"=6.7380595, "y"=6.075366, "Z"=-5.890599e-07}, {"x"=6.7583523, "y"=6.0273914, "Z"=-5.908339e-07}, {"x"=6.7743764, "y"=5.976284, "Z"=-5.922348e-07}, {"x"=6.805071, "y"=5.936787, "Z"=-5.9491816e-07}, {"x"=6.807713, "y"=5.875877, "Z"=-5.951492e-07}, {"x"=6.834629, "y"=5.8337793, "Z"=-5.9750226e-07}, {"x"=6.8364263, "y"=5.773024, "Z"=-5.976594e-07}, {"x"=6.8280845, "y"=5.7053103, "Z"=-5.969301e-07}, {"x"=6.8183784, "y"=5.637279, "Z"=-5.960816e-07}, {"x"=6.824358, "y"=5.581198, "Z"=-5.966043e-07}, {"x"=6.8486753, "y"=5.5385237, "Z"=-5.987302e-07}, {"x"=6.840788, "y"=5.4733524, "Z"=-5.980407e-07}, {"x"=6.846354, "y"=5.4181128, "Z"=-5.9852727e-07}, {"x"=6.83087, "y"=5.3488636, "Z"=-5.9717365e-07}, {"x"=6.8380218, "y"=5.295621, "Z"=-5.977989e-07}, {"x"=6.8081737, "y"=5.2180495, "Z"=-5.951894e-07}, {"x"=6.834457, "y"=5.178369, "Z"=-5.974872e-07}, {"x"=5.3789005, "y"=4.175662, "Z"=-4.7023843e-07}, {"x"=5.3940945, "y"=4.1410728, "Z"=-4.7156672e-07}, {"x"=5.5298705, "y"=4.1829486, "Z"=-4.834366e-07}, {"x"=6.9839015, "y"=5.0472975, "Z"=-6.1055204e-07}, {"x"=6.9955735, "y"=4.9981933, "Z"=-6.115725e-07}, {"x"=7.009473, "y"=4.9506617, "Z"=-6.127876e-07}, {"x"=5.7307115, "y"=4.126, "Z"=-5.009947e-07}, {"x"=5.9260955, "y"=4.1967134, "Z"=-5.180757e-07}, {"x"=0.0, "y"=0.68, "Z"=0.0}, {"x"=6.677475, "y"=4.538273, "Z"=-5.837634e-07}, {"x"=6.6329126, "y"=4.4612293, "Z"=-5.798676e-07}, {"x"=6.657411, "y"=4.4240513, "Z"=-5.8200936e-07}, {"x"=6.6204896, "y"=4.3527584, "Z"=-5.7878157e-07}, {"x"=6.6075296, "y"=4.2954636, "Z"=-5.7764856e-07}, {"x"=6.6134887, "y"=4.248892, "Z"=-5.7816953e-07}, {"x"=6.591764, "y"=4.187811, "Z"=-5.762703e-07}, {"x"=6.5704393, "y"=4.1275682, "Z"=-5.7440604e-07}, {"x"=6.549526, "y"=4.068153, "Z"=-5.725778e-07}, {"x"=6.5477443, "y"=4.019093, "Z"=-5.72422e-07}, {"x"=6.53936, "y"=3.967025, "Z"=-5.71689e-07}, {"x"=6.5494094, "y"=3.92449, "Z"=-5.7256756e-07}, {"x"=6.5501995, "y"=3.8775625, "Z"=-5.726366e-07}, {"x"=6.565085, "y"=3.8376713, "Z"=-5.7393794e-07}, {"x"=6.5896683, "y"=3.8024251, "Z"=-5.760871e-07}, {"x"=6.591409, "y"=3.7564263, "Z"=-5.762393e-07}, {"x"=6.62464, "y"=3.7251313, "Z"=-5.791444e-07}, {"x"=6.638598, "y"=3.6848936, "Z"=-5.8036466e-07}, {"x"=6.6258235, "y"=3.6327922, "Z"=-5.792479e-07}, {"x"=6.641972, "y"=3.5937972, "Z"=-5.806596e-07}, {"x"=6.623005, "y"=3.539651, "Z"=-5.790015e-07}, {"x"=6.653333, "y"=3.5069413, "Z"=-5.8165284e-07}, {"x"=6.695499, "y"=3.4789894, "Z"=-5.853391e-07}, {"x"=6.711668, "y"=3.4399934, "Z"=-5.8675266e-07}, {"x"=6.7081413, "y"=3.3930302, "Z"=-5.8644434e-07}, {"x"=6.731244, "y"=3.3569183, "Z"=-5.8846405e-07}, {"x"=6.760672, "y"=3.3231783, "Z"=-5.910367e-07}, {"x"=6.7778006, "y"=3.2845232, "Z"=-5.9253415e-07}, {"x"=6.7741265, "y"=3.2379863, "Z"=-5.922129e-07}, {"x"=6.7776413, "y"=3.194363, "Z"=-5.925202e-07}, {"x"=6.7780595, "y"=3.1497586, "Z"=-5.925568e-07}, {"x"=6.8214993, "y"=3.1207314, "Z"=-5.963544e-07}, {"x"=6.8157687, "y"=3.074049, "Z"=-5.958534e-07}, {"x"=6.8295803, "y"=3.0343602, "Z"=-5.970609e-07}, {"x"=6.8545275, "y"=2.9984365, "Z"=-5.9924184e-07}, {"x"=6.8821354, "y"=2.9632466, "Z"=-6.0165536e-07}, {"x"=6.8658214, "y"=2.9135835, "Z"=-6.0022916e-07}, {"x"=6.869171, "y"=2.8705678, "Z"=-6.00522e-07}, {"x"=6.8951607, "y"=2.8347478, "Z"=-6.027941e-07}, {"x"=6.913316, "y"=2.7963574, "Z"=-6.043813e-07}, {"x"=6.890068, "y"=2.7454813, "Z"=-6.023489e-07}, {"x"=6.8664637, "y"=2.6949475, "Z"=-6.002853e-07}, {"x"=6.8723016, "y"=2.653314, "Z"=-6.0079566e-07}, {"x"=6.8682604, "y"=2.6089773, "Z"=-6.004424e-07}, {"x"=6.8909373, "y"=2.5721684, "Z"=-6.0242485e-07}, {"x"=6.876716, "y"=2.5253122, "Z"=-6.011816e-07}, {"x"=6.8844323, "y"=2.4845173, "Z"=-6.018562e-07}, {"x"=6.893844, "y"=2.4441912, "Z"=-6.02679e-07}, {"x"=6.901079, "y"=2.403332, "Z"=-6.033115e-07}, {"x"=6.873095, "y"=2.3539295, "Z"=-6.0086506e-07}, {"x"=6.822393, "y"=2.299599, "Z"=-5.964325e-07}, {"x"=6.825853, "y"=2.2585328, "Z"=-5.96735e-07}, {"x"=6.577367, "y"=2.160814, "Z"=-5.7501165e-07}, {"x"=6.1912255, "y"=2.036087, "Z"=-5.412541e-07}, {"x"=6.140325, "y"=1.9875524, "Z"=-5.368043e-07}, {"x"=6.061652, "y"=1.9339838, "Z"=-5.2992647e-07}, {"x"=5.9855075, "y"=1.8819661, "Z"=-5.232697e-07}, {"x"=5.9629517, "y"=1.8413918, "Z"=-5.212978e-07}, {"x"=5.924405, "y"=1.7981536, "Z"=-5.1792796e-07}, {"x"=5.900314, "y"=1.7580996, "Z"=-5.158218e-07}, {"x"=5.8651266, "y"=1.7164495, "Z"=-5.1274566e-07}, {"x"=5.8631706, "y"=1.6809673, "Z"=-5.125747e-07}, {"x"=5.856067, "y"=1.6447303, "Z"=-5.1195366e-07}, {"x"=5.8161488, "y"=1.6034353, "Z"=-5.0846387e-07}, {"x"=5.7838583, "y"=1.563846, "Z"=-5.0564097e-07}, {"x"=5.7651567, "y"=1.5266981, "Z"=-5.04006e-07}, {"x"=5.746219, "y"=1.4897978, "Z"=-5.023504e-07}, {"x"=5.7438955, "y"=1.455421, "Z"=-5.021473e-07}, {"x"=5.739383, "y"=1.4208426, "Z"=-5.017528e-07}, {"x"=5.7326784, "y"=1.3860986, "Z"=-5.0116665e-07}, {"x"=5.721791, "y"=1.3509917, "Z"=-5.002148e-07}, {"x"=5.727585, "y"=1.3179172, "Z"=-5.0072134e-07}, {"x"=5.7302046, "y"=1.2844833, "Z"=-5.009504e-07}, {"x"=5.722678, "y"=1.2500494, "Z"=-5.002924e-07}, {"x"=5.7249017, "y"=1.2166567, "Z"=-5.004868e-07}, {"x"=5.7249384, "y"=1.1830823, "Z"=-5.0049e-07}, {"x"=5.718798, "y"=1.1490353, "Z"=-4.999532e-07}, {"x"=5.715447, "y"=1.1153046, "Z"=-4.9966025e-07}, {"x"=5.703917, "y"=1.0810677, "Z"=-4.9865224e-07}, {"x"=5.697172, "y"=1.0473013, "Z"=-4.980626e-07}, {"x"=5.698214, "y"=1.0140953, "Z"=-4.9815367e-07}, {"x"=5.685082, "y"=0.9801514, "Z"=-4.9700566e-07}, {"x"=5.6837354, "y"=0.9469346, "Z"=-4.9688794e-07}, {"x"=5.691187, "y"=0.9141135, "Z"=-4.9753936e-07}, {"x"=5.7054443, "y"=0.88146186, "Z"=-4.9878577e-07}, {"x"=5.7245116, "y"=0.8487996, "Z"=-5.004527e-07}, {"x"=5.7303953, "y"=0.81561464, "Z"=-5.009671e-07}, {"x"=5.738086, "y"=0.7824027, "Z"=-5.016394e-07}, {"x"=5.7465844, "y"=0.74911785, "Z"=-5.0238236e-07}, {"x"=5.7328897, "y"=0.715601, "Z"=-5.011851e-07}, {"x"=5.7479997, "y"=0.68225724, "Z"=-5.025061e-07}, {"x"=5.7589154, "y"=0.64876056, "Z"=-5.034604e-07}, {"x"=5.7626357, "y"=0.61521566, "Z"=-5.037856e-07}, {"x"=5.7891574, "y"=0.5812341, "Z"=-5.061042e-07}, {"x"=5.7914844, "y"=0.5474907, "Z"=-5.0630763e-07}, {"x"=5.8036103, "y"=0.51343006, "Z"=-5.073677e-07}, {"x"=5.827528, "y"=0.47880983, "Z"=-5.094587e-07}, {"x"=5.83725, "y"=0.44447017, "Z"=-5.103086e-07}, {"x"=5.8627524, "y"=0.40927252, "Z"=-5.125381e-07}, {"x"=5.886045, "y"=0.37387413, "Z"=-5.1457437e-07}, {"x"=5.8841643, "y"=0.3396393, "Z"=-5.1441e-07}, {"x"=5.886077, "y"=0.30516177, "Z"=-5.145772e-07}, {"x"=5.9017534, "y"=0.2696795, "Z"=-5.1594765e-07}, {"x"=5.9521165, "y"=0.23137158, "Z"=-5.2035057e-07}, {"x"=5.9832945, "y"=0.19400221, "Z"=-5.230762e-07}, {"x"=6.0112495, "y"=0.1565153, "Z"=-5.2552014e-07}, {"x"=6.0728235, "y"=0.11554009, "Z"=-5.309031e-07}, {"x"=6.1450686, "y"=0.07274926, "Z"=-5.3721897e-07}, {"x"=6.2926064, "y"=0.021185338, "Z"=-5.5011714e-07}, {"x"=6.47851, "y"=-0.03640157, "Z"=-5.6636935e-07}, {"x"=6.6977224, "y"=-0.10010648, "Z"=-5.855335e-07}, {"x"=6.8042417, "y"=-0.15265924, "Z"=-5.948457e-07}, {"x"=6.8369737, "y"=-0.19706154, "Z"=-5.9770724e-07}, {"x"=6.8377028, "y"=-0.23761648, "Z"=-5.9777096e-07}, {"x"=6.857998, "y"=-0.28098494, "Z"=-5.995452e-07}, {"x"=6.873071, "y"=-0.32389778, "Z"=-6.0086296e-07}, {"x"=6.8928194, "y"=-0.36776978, "Z"=-6.025894e-07}, {"x"=6.914265, "y"=-0.41221756, "Z"=-6.044643e-07}, {"x"=6.9176626, "y"=-0.45403808, "Z"=-6.047613e-07}, {"x"=6.9306664, "y"=-0.49761027, "Z"=-6.058981e-07}, {"x"=6.937487, "y"=-0.5403324, "Z"=-6.064944e-07}, {"x"=6.2287827, "y"=-0.45306224, "Z"=-5.445375e-07}, {"x"=6.1572213, "y"=-0.4770872, "Z"=-5.3828137e-07}, {"x"=6.1513677, "y"=-0.51307553, "Z"=-5.3776967e-07}, {"x"=6.1580515, "y"=-0.5515843, "Z"=-5.3835396e-07}, {"x"=8.640479, "y"=-1.1003945, "Z"=-7.553747e-07}, {"x"=6.966001, "y"=-0.7976578, "Z"=-6.0898714e-07}, {"x"=6.9729195, "y"=-0.84156615, "Z"=-6.09592e-07}, {"x"=6.9776106, "y"=-0.8851672, "Z"=-6.100021e-07}, {"x"=6.977158, "y"=-0.9277515, "Z"=-6.099625e-07}, {"x"=6.9822845, "y"=-0.9717646, "Z"=-6.104107e-07}, {"x"=6.9745016, "y"=-1.0128253, "Z"=-6.097303e-07}, {"x"=6.957743, "y"=-1.051678, "Z"=-6.082652e-07}, {"x"=6.958211, "y"=-1.0948415, "Z"=-6.083061e-07}, {"x"=6.9758267, "y"=-1.1426194, "Z"=-6.0984615e-07}, {"x"=6.9815288, "y"=-1.187561, "Z"=-6.103446e-07}, {"x"=6.9618664, "y"=-1.2257657, "Z"=-6.0862567e-07}, {"x"=6.9660697, "y"=-1.270546, "Z"=-6.0899316e-07}, {"x"=6.9478755, "y"=-1.309109, "Z"=-6.0740257e-07}, {"x"=6.9323483, "y"=-1.3483686, "Z"=-6.0604515e-07}, {"x"=6.935761, "y"=-1.3932433, "Z"=-6.0634346e-07}, {"x"=6.941756, "y"=-1.4391019, "Z"=-6.0686756e-07}, {"x"=6.918809, "y"=-1.4761746, "Z"=-6.048615e-07}, {"x"=6.8680305, "y"=-1.5042629, "Z"=-6.004223e-07}, {"x"=6.8761344, "y"=-1.5509677, "Z"=-6.0113075e-07}, {"x"=6.8744326, "y"=-1.5946991, "Z"=-6.00982e-07}, {"x"=6.871507, "y"=-1.6381664, "Z"=-6.0072625e-07}, {"x"=6.815351, "y"=-1.6634674, "Z"=-5.958169e-07}, {"x"=6.59681, "y"=-1.6313202, "Z"=-5.7671144e-07}, {"x"=6.3835893, "y"=-1.598393, "Z"=-5.580711e-07}, {"x"=6.7010508, "y"=-1.7557383, "Z"=-5.8582447e-07}, {"x"=6.847138, "y"=-1.8540287, "Z"=-5.985958e-07}, {"x"=6.8350887, "y"=-1.8948743, "Z"=-5.9754245e-07}, {"x"=6.8199944, "y"=-1.9345915, "Z"=-5.9622283e-07}, {"x"=6.8829274, "y"=-2.0047452, "Z"=-6.0172465e-07}, {"x"=5.8047676, "y"=-1.6231935, "Z"=-5.074689e-07}, {"x"=5.58911, "y"=-1.5753446, "Z"=-4.886155e-07}, {"x"=6.824852, "y"=-2.1202724, "Z"=-5.966475e-07}, {"x"=6.8259826, "y"=-2.1672406, "Z"=-5.9674636e-07}, {"x"=6.821273, "y"=-2.2119746, "Z"=-5.963346e-07}, {"x"=6.813518, "y"=-2.2555628, "Z"=-5.956567e-07}, {"x"=6.7981586, "y"=-2.2959504, "Z"=-5.943139e-07}, {"x"=6.801748, "y"=-2.344792, "Z"=-5.946277e-07}, {"x"=6.8332496, "y"=-2.4065363, "Z"=-5.9738164e-07}, {"x"=6.8069983, "y"=-2.4424818, "Z"=-5.950867e-07}, {"x"=6.766057, "y"=-2.4714706, "Z"=-5.915075e-07}, {"x"=6.8108916, "y"=-2.5407007, "Z"=-5.954271e-07}, {"x"=6.7514725, "y"=-2.560793, "Z"=-5.9023245e-07}, {"x"=6.8206067, "y"=-2.642934, "Z"=-5.962764e-07}, {"x"=0.0, "y"=0.68, "Z"=0.0}, {"x"=0.0017876594, "y"=0.6791032, "Z"=-1.5628214e-10}, {"x"=7.081524, "y"=-2.9242942, "Z"=-6.190865e-07}, {"x"=6.786763, "y"=-2.8241248, "Z"=-5.933177e-07}, {"x"=6.6900797, "y"=-2.8236465, "Z"=-5.8486535e-07}, {"x"=6.6157126, "y"=-2.8338904, "Z"=-5.78364e-07}, {"x"=6.5872364, "y"=-2.8680477, "Z"=-5.758745e-07}, {"x"=6.605101, "y"=-2.9273968, "Z"=-5.7743625e-07}, {"x"=6.61025, "y"=-2.9802914, "Z"=-5.778864e-07}, {"x"=6.6228538, "y"=-3.037773, "Z"=-5.7898825e-07}, {"x"=6.6706457, "y"=-3.1158013, "Z"=-5.8316635e-07}, {"x"=6.5990763, "y"=-3.1260633, "Z"=-5.7690954e-07}, {"x"=6.5017147, "y"=-3.1204827, "Z"=-5.68398e-07}, {"x"=6.4657307, "y"=-3.1500852, "Z"=-5.6525215e-07}, {"x"=5.001199, "y"=-2.3219829, "Z"=-4.372187e-07}, {"x"=4.954602, "y"=-2.333357, "Z"=-4.3314503e-07}, {"x"=4.9574213, "y"=-2.3747182, "Z"=-4.3339153e-07}, {"x"=0.0016965714, "y"=0.67894095, "Z"=-1.4831898e-10}, {"x"=0.31525624, "y"=0.48064476, "Z"=-2.7560576e-08}, {"x"=0.31324914, "y"=0.4793536, "Z"=-2.738511e-08}, {"x"=0.30452642, "y"=0.48243314, "Z"=-2.6622544e-08}, {"x"=0.29752183, "y"=0.48450893, "Z"=-2.6010184e-08}, {"x"=0.2963796, "y"=0.48278153, "Z"=-2.5910326e-08}, {"x"=0.29771522, "y"=0.4793843, "Z"=-2.6027092e-08}, {"x"=0.29571712, "y"=0.4782195, "Z"=-2.5852412e-08}, {"x"=0.29207015, "y"=0.47820795, "Z"=-2.5533584e-08}, {"x"=0.2933496, "y"=0.47479272, "Z"=-2.5645436e-08}, {"x"=0.2872545, "y"=0.47655752, "Z"=-2.5112588e-08}, {"x"=0.28444082, "y"=0.47605535, "Z"=-2.4866607e-08}, {"x"=0.2735382, "y"=0.48145318, "Z"=-2.3913469e-08}, {"x"=0.2747962, "y"=0.47808897, "Z"=-2.4023446e-08}, {"x"=0.27361697, "y"=0.47649387, "Z"=-2.3920355e-08}, {"x"=0.27482525, "y"=0.4731013, "Z"=-2.4025987e-08}, {"x"=0.26884466, "y"=0.4751426, "Z"=-2.3503148e-08}, {"x"=0.26764843, "y"=0.47358215, "Z"=-2.3398568e-08}, {"x"=0.26407826, "y"=0.47387463, "Z"=-2.3086455e-08}, {"x"=0.2644441, "y"=0.47110218, "Z"=-2.3118439e-08}, {"x"=0.26088122, "y"=0.47144067, "Z"=-2.280696e-08}, {"x"=0.25499895, "y"=0.4737004, "Z"=-2.2292717e-08}, {"x"=0.24915199, "y"=0.47602135, "Z"=-2.1781558e-08}, {"x"=0.2479612, "y"=0.47457546, "Z"=-2.1677456e-08}, {"x"=0.24446298, "y"=0.4750638, "Z"=-2.1371633e-08}, {"x"=0.2432667, "y"=0.4736452, "Z"=-2.126705e-08}, {"x"=0.24054456, "y"=0.4735362, "Z"=-2.1029074e-08}, {"x"=0.2408495, "y"=0.47082895, "Z"=-2.1055731e-08}, {"x"=0.24338457, "y"=0.466131, "Z"=-2.1277355e-08}, {"x"=0.24512568, "y"=0.46206105, "Z"=-2.1429567e-08}, {"x"=0.24608412, "y"=0.4586324, "Z"=-2.1513358e-08}, {"x"=0.24035491, "y"=0.46124327, "Z"=-2.1012493e-08}, {"x"=0.24569893, "y"=0.45375228, "Z"=-2.1479682e-08}, {"x"=0.24291532, "y"=0.45369017, "Z"=-2.1236332e-08}, {"x"=0.23868394, "y"=0.4550245, "Z"=-2.0866413e-08}, {"x"=0.24171335, "y"=0.44949913, "Z"=-2.1131251e-08}, {"x"=0.2425274, "y"=0.446014, "Z"=-2.1202418e-08}, {"x"=0.23973092, "y"=0.4460041, "Z"=-2.0957943e-08}, {"x"=0.24121185, "y"=0.44180292, "Z"=-2.108741e-08}, {"x"=0.23628493, "y"=0.44393766, "Z"=-2.0656683e-08}], 11 "raw data in":string="\u0002sRA LMDscandata 1 1 127E169 0 0 469E 46A0 4D0BFA83 4D0C0E59 0 0 1 0 0 5DC A2 0 1 DIST1 3F800000 00000000 FFF92230 D05 32B 14E 14B 14A 14F 14D 148 146 141 13D 14B 146 146 14A 145 149 140 142 152 143 152 150 150 2 150 155 15C 157 15C 159 159 15B 164 167 175 177 16E 17A 17A 17B 180 18A 18ED 18D4 18BE 18B5 18B0 18A2 1891 188B 187E 187F 187B 186F 1861 1855 1845 184A 1841 183E 1840 184F 185B 185C 184E 184F 184E 185C 1867 1861 185A 1871 1880 188E 1893 188C 1890 1880 186F 1851 183B 181A 17F7 17F6 1819 1852 183F 1828 180A 1821 1879 18C3 1871 17C3 17D4 1784 1793 17AC 17AC 17CF 17F3 17CD 17D8 17FC 1821 1824 17E5 17A7 179F 178D 177D 179F 1795 1785 1752 170C 1718 1726 1709 16ED 16DB 16E0 16D4 16E0 16F5 1754 1762 1749 1728 1740 1738 1733 1735 1734 172B 1722 16FD 16F7 16FA 170E 1730 174F 1777 1780 176C 1745 1745 1740 1740 1742 1738 1736 170D 1717 171C 171A 1718 1735 1744 1760 1767 1760 1757 1761 1771 1796 17A0 17AB 17AC 179F 17B9 17BE 17D0 17E2 17FC 181B 1829 181A 1826 17FC 17D1 17CB 17E8 180A 1815 1816 182C 1858 1878 188E 1896 18D1 18DA 18D7 18EC 1907 1906 1921 1927 1948 1956 198B 19C0 19AC 19C2 19ED 1A06 1A02 1A0B 1A27 1A4E 1A5D 1A59 1A6B 1A7E 1AB2 1ABF 1AB1 1ABD 1AC9 1AF1 1B24 1B55 1BB2 1CC0 1D91 1DC4 1DBF 1DAF 1DCA 1DB5 1DBF 1D6D 1D4C 1D49 1D0E 1CE6 1CD4 1CBB 1CBA 2 1ECD 1F22 1F2C 1F59 0 222A 222F 2268 2288 22AF 22FE 2388 243B 2428 2449 244E 244F 244B 24A5 24AA 249E 253E 25F9 263F 268C 265E 25E6 25F7 25ED 25A3 25C4 25F0 2583 2572 2640 266A 0 0 0 0 0 0 0 0 0 0 2869 2887 28A5 0 0 0 0 0 0 0 0 0 0 0 0 0 2AF9 0 0 0 0 0 0 0 0 0 0 0 0 0 0 0 0 0 0 0 0 0 0 0 0 0 0 0 0 0 0 0 0 0 0 0 0 0 0 0 0 0 0 0 0 0 0 0 0 0 0 0 0 0 0 0 0 0 0 0 0 0 0 0 0 0 0 0 0 0 0 0 0 0 0 0 0 0 0 0 0 0 0 0 0 0 0 0 0 0 0 0 0 0 0 0 0 0 0 0 0 0 0 0 0 0 0 0 0 0 0 0 0 0 0 0 0 0 0 0 0 0 0 0 0 0 0 0 0 0 0 0 0 0 0 0 0 0 0 0 0 0 0 0 0 0 0 0 0 0 0 0 0 0 0 0 0 0 0 0 0 0 0 0 0 0 0 0 0 0 0 0 0 0 0 0 0 0 0 0 0 0 0 0 0 0 0 0 0 0 0 0 0 0 0 0 0 0 2793 2777 2756 0 0 0 29C1 29EF 2A44 2A2A 2937 2881 297F 2AAB 2AA7 0 265C 253C 2431 2436 24A9 2477 2427 2439 2423 2498 24C4 2510 2564 259E 2626 2621 26C1 279B 287E 28DE 0 294E 2921 2910 28E9 28DC 0 0 0 0 2399 23E7 2 246B 24A8 1DF6 1DAA 23DF 239D 22D8 2247 21D2 21D2 21B8 21AA 2197 2197 2174 2170 214D 211E 20EE 20D2 20CD 20A1 2086 2052 203A 1FF6 1FF6 190F 1909 1992 202D 201D 2010 1A1F 1AEB 0 1E20 1DD3 1DD6 1D93 1D6C 1D5B 1D2B 1CFC 1CCE 1CB6 1C97 1C8D 1C79 1C75 1C7C 1C6A 1C7B 1C77 1C56 1C55 1C2E 1C3D 1C59 1C59 1C44 1C4C 1C5B 1C5D 1C49 1C3D 1C2E 1C4D 1C38 1C38 1C44 1C53 1C34 1C2A 1C38 1C3E 1C19 1BF4 1BEE 1BDE 1BEA 1BD0 1BCD 1BCC 1BC9 1BA2 1B64 1B5E 1A56 18C2 1886 182E 17D9 17BB 178D 176E 1744 173C 172F 1701 16DB 16C3 16AB 16A4 169B 1690 1681 1683 1682 1677 1676 1673 166A 1664 1656 164D 164C 163D 163A 1640 164D 165F 1664 166B 1673 1665 1674 167F 1683 169E 16A1 16AE 16C7 16D2 16ED 1706 1706 170A 171C 1751 1773 1792 17D3 181F 18B7 1976 1A57 1AC7 1AED 1AF3 1B0D 1B22 1B3C 1B58 1B62 1B76 1B84 18BB 1879 187A 1888 2276 1BD1 1BE1 1BEF 1BF8 1C07 1C09 1C02 1C0D 1C2A 1C3B 1C32 1C42 1C3B 1C37 1C47 1C5A 1C4F 1C27 1C3D 1C49 1C54 1C27 1B4E 1A7A 1BDA 1C85 1C88 1C88 1CDC 1865 178B 1CD1 1CE4 1CF1 1CFB 1CFD 1D14 1D4A 1D41 1D28 1D6E 1D41 1DA3 0 2 1F0A 1DD6 1D80 1D43 1D3A 1D66 1D84 1DAB 1DFB 1DC2 1D6B 1D5B 16C9 16A7 16BF 2 175 174 16B 164 164 167 166 163 166 160 15E 152 155 155 158 152 152 14F 151 14E 148 142 142 13F 13F 13D 13F 144 148 14B 145 14E 14C 148 14E 151 14F 153 14E 0 0 1 B not defined 0 0 0\u0003") -> (0 "error out":errorcluster, 2 "XYZ_DATA out":cluster{"x":sgl, "y":sgl, "Z":sgl}[](array[cluster])=[{"x"=-0.23617366, "y"=0.44382635, "Z"=2.0646958e-08}, {"x"=-0.2354099, "y"=0.44731313, "Z"=2.0580186e-08}, {"x"=-0.23604421, "y"=0.44938534, "Z"=2.063564e-08}, {"x"=-0.24097842, "y"=0.44728905, "Z"=2.1067002e-08}, {"x"=-0.24088132, "y"=0.4500757, "Z"=2.1058515e-08}, {"x"=-0.2385779, "y"=0.45491207, "Z"=2.0857142e-08}, {"x"=-0.23842053, "y"=0.4576677, "Z"=2.0843386e-08}, {"x"=-0.2360333, "y"=0.46244708, "Z"=2.0634687e-08}, {"x"=-0.23433791, "y"=0.46651757, "Z"=2.0486471e-08}, {"x"=-0.24597977, "y"=0.45851648, "Z"=2.1504235e-08}, {"x"=-0.24352892, "y"=0.46327513, "Z"=2.1289974e-08}, {"x"=-0.24478552, "y"=0.46469545, "Z"=2.139983e-08}, {"x"=-0.24905264, "y"=0.46349877, "Z"=2.1772873e-08}, {"x"=-0.24651532, "y"=0.46820956, "Z"=2.1551054e-08}, {"x"=-0.2507923, "y"=0.46705818, "Z"=2.192496e-08}, {"x"=-0.24513243, "y"=0.47430584, "Z"=2.1430157e-08}, {"x"=-0.24786437, "y"=0.47445863, "Z"=2.1668992e-08}, {"x"=-0.26143128, "y"=0.46576256, "Z"=2.2855048e-08}, {"x"=-0.25101602, "y"=0.4767269, "Z"=2.1944517e-08}, {"x"=-0.26390603, "y"=0.46881858, "Z"=2.3071397e-08}, {"x"=-0.26356125, "y"=0.47159782, "Z"=2.3041256e-08}, {"x"=-0.26476908, "y"=0.47313452, "Z"=2.3146848e-08}, {"x"=-0.0015831427, "y"=0.6787779, "Z"=1.3840273e-10}, {"x"=-0.26715785, "y"=0.47622886, "Z"=2.3355682e-08}, {"x"=-0.27233183, "y"=0.47477728, "Z"=2.3808004e-08}, {"x"=-0.27913585, "y"=0.47218478, "Z"=2.4402832e-08}, {"x"=-0.27631214, "y"=0.4767745, "Z"=2.4155975e-08}, {"x"=-0.2815347, "y"=0.4754463, "Z"=2.4612545e-08}, {"x"=-0.28028262, "y"=0.47883677, "Z"=2.4503084e-08}, {"x"=-0.28144807, "y"=0.4804706, "Z"=2.4604972e-08}, {"x"=-0.28424227, "y"=0.480964, "Z"=2.4849248e-08}, {"x"=-0.29279748, "y"=0.4775015, "Z"=2.5597169e-08}, {"x"=-0.29644778, "y"=0.4775161, "Z"=2.5916288e-08}, {"x"=-0.30922702, "y"=0.4714151, "Z"=2.7033485e-08}, {"x"=-0.31209967, "y"=0.47210872, "Z"=2.7284619e-08}, {"x"=-0.30578443, "y"=0.4788735, "Z"=2.6732524e-08}, {"x"=-0.31701317, "y"=0.4741198, "Z"=2.7714172e-08}, {"x"=-0.31820545, "y"=0.4759674, "Z"=2.7818404e-08}, {"x"=-0.32023188, "y"=0.47728705, "Z"=2.799556e-08}, {"x"=-0.32564586, "y"=0.4765036, "Z"=2.8468866e-08}, {"x"=-0.33533517, "y"=0.47315145, "Z"=2.9315931e-08}, {"x"=-5.450293, "y"=-2.6383529, "Z"=4.7647976e-07}, {"x"=-5.4480753, "y"=-2.593715, "Z"=4.7628586e-07}, {"x"=-5.448104, "y"=-2.550746, "Z"=4.7628836e-07}, {"x"=-5.459038, "y"=-2.5144534, "Z"=4.772442e-07}, {"x"=-5.473198, "y"=-2.4801433, "Z"=4.7848215e-07}, {"x"=-5.4793234, "y"=-2.4413216, "Z"=4.790177e-07}, {"x"=-5.482568, "y"=-2.4010663, "Z"=4.793013e-07}, {"x"=-5.4951506, "y"=-2.3662121, "Z"=4.804013e-07}, {"x"=-5.5013714, "y"=-2.3279579, "Z"=4.809452e-07}, {"x"=-5.519656, "y"=-2.2963793, "Z"=4.8254367e-07}, {"x"=-5.533345, "y"=-2.2623425, "Z"=4.837404e-07}, {"x"=-5.53974, "y"=-2.2245321, "Z"=4.8429945e-07}, {"x"=-5.5441055, "y"=-2.1858287, "Z"=4.846811e-07}, {"x"=-5.5499907, "y"=-2.148081, "Z"=4.851956e-07}, {"x"=-5.5520506, "y"=-2.108567, "Z"=4.8537566e-07}, {"x"=-5.572659, "y"=-2.0784407, "Z"=4.871773e-07}, {"x"=-5.580522, "y"=-2.0420315, "Z"=4.878647e-07}, {"x"=-5.593558, "y"=-2.008223, "Z"=4.890044e-07}, {"x"=-5.610909, "y"=-1.976495, "Z"=4.9052124e-07}, {"x"=-5.6398616, "y"=-1.9501503, "Z"=4.9305237e-07}, {"x"=-5.665971, "y"=-1.9223063, "Z"=4.953349e-07}, {"x"=-5.6819243, "y"=-1.8897145, "Z"=4.967296e-07}, {"x"=-5.683987, "y"=-1.8509235, "Z"=4.9690993e-07}, {"x"=-5.6995296, "y"=-1.8182178, "Z"=4.982687e-07}, {"x"=-5.7130475, "y"=-1.7846243, "Z"=4.994505e-07}, {"x"=-5.740175, "y"=-1.7568197, "Z"=5.01822e-07}, {"x"=-5.7644033, "y"=-1.7276263, "Z"=5.0394016e-07}, {"x"=-5.7727613, "y"=-1.6917732, "Z"=5.046708e-07}, {"x"=-5.77997, "y"=-1.6555295, "Z"=5.0530105e-07}, {"x"=-5.814833, "y"=-1.6303596, "Z"=5.083489e-07}, {"x"=-5.842147, "y"=-1.6019523, "Z"=5.107367e-07}, {"x"=-5.868392, "y"=-1.5729468, "Z"=5.130311e-07}, {"x"=-5.886077, "y"=-1.5405362, "Z"=5.145772e-07}, {"x"=-5.8923306, "y"=-1.5038257, "Z"=5.1512393e-07}, {"x"=-5.9086933, "y"=-1.4708805, "Z"=5.165544e-07}, {"x"=-5.9060388, "y"=-1.4310868, "Z"=5.163223e-07}, {"x"=-5.9021783, "y"=-1.3910661, "Z"=5.159848e-07}, {"x"=-5.8857613, "y"=-1.3469288, "Z"=5.145496e-07}, {"x"=-5.8766103, "y"=-1.305614, "Z"=5.1374957e-07}, {"x"=-5.8567367, "y"=-1.2610137, "Z"=5.120122e-07}, {"x"=-5.8346424, "y"=-1.2160943, "Z"=5.1008067e-07}, {"x"=-5.8446207, "y"=-1.1818175, "Z"=5.10953e-07}, {"x"=-5.8887625, "y"=-1.1582162, "Z"=5.14812e-07}, {"x"=-5.9538646, "y"=-1.1405971, "Z"=5.2050336e-07}, {"x"=-5.9461527, "y"=-1.1004817, "Z"=5.198292e-07}, {"x"=-5.934338, "y"=-1.0593927, "Z"=5.187963e-07}, {"x"=-5.9155188, "y"=-1.0165718, "Z"=5.171511e-07}, {"x"=-5.947433, "y"=-0.98834354, "Z"=5.199411e-07}, {"x"=-6.0419035, "y"=-0.9769929, "Z"=5.2819996e-07}, {"x"=-6.122918, "y"=-0.9609745, "Z"=5.352825e-07}, {"x"=-6.0530334, "y"=-0.90456265, "Z"=5.29173e-07}, {"x"=-5.893567, "y"=-0.8262395, "Z"=5.15232e-07}, {"x"=-5.918724, "y"=-0.7960438, "Z"=5.174313e-07}, {"x"=-5.8494763, "y"=-0.74268264, "Z"=5.1137744e-07}, {"x"=-5.8722486, "y"=-0.7120914, "Z"=5.1336826e-07}, {"x"=-5.9046063, "y"=-0.68353313, "Z"=5.161971e-07}, {"x"=-5.9124384, "y"=-0.6491621, "Z"=5.1688176e-07}, {"x"=-5.9542623, "y"=-0.62222403, "Z"=5.2053815e-07}, {"x"=-5.9969497, "y"=-0.59505194, "Z"=5.2427e-07}, {"x"=-5.9670506, "y"=-0.5524588, "Z"=5.2165615e-07}, {"x"=-5.984905, "y"=-0.51988906, "Z"=5.23217e-07}, {"x"=-6.0271215, "y"=-0.49192494, "Z"=5.269077e-07}, {"x"=-6.070197, "y"=-0.4636951, "Z"=5.306735e-07}, {"x"=-6.0796986, "y"=-0.4289028, "Z"=5.3150416e-07}, {"x"=-6.024004, "y"=-0.3825739, "Z"=5.266352e-07}, {"x"=-5.968964, "y"=-0.33709878, "Z"=5.2182344e-07}, {"x"=-5.966886, "y"=-0.30106133, "Z"=5.2164177e-07}, {"x"=-5.954714, "y"=-0.26351756, "Z"=5.205776e-07}, {"x"=-5.9442844, "y"=-0.22645015, "Z"=5.1966583e-07}, {"x"=-5.9830976, "y"=-0.19678587, "Z"=5.23059e-07}, {"x"=-5.978194, "y"=-0.16057408, "Z"=5.2263033e-07}, {"x"=-5.967126, "y"=-0.123648226, "Z"=5.2166274e-07}, {"x"=-5.9211173, "y"=-0.08240992, "Z"=5.176405e-07}, {"x"=-5.8559747, "y"=-0.039417505, "Z"=5.119456e-07}, {"x"=-5.871979, "y"=-0.0067341924, "Z"=5.1334473e-07}, {"x"=-5.889789, "y"=0.02589035, "Z"=5.149017e-07}, {"x"=-5.8646536, "y"=0.06319648, "Z"=5.127043e-07}, {"x"=-5.8402796, "y"=0.10008913, "Z"=5.1057344e-07}, {"x"=-5.825632, "y"=0.13574708, "Z"=5.0929293e-07}, {"x"=-5.8336806, "y"=0.1692087, "Z"=5.0999654e-07}, {"x"=-5.824593, "y"=0.20412987, "Z"=5.092021e-07}, {"x"=-5.839228, "y"=0.23711291, "Z"=5.104815e-07}, {"x"=-5.8626547, "y"=0.2696217, "Z"=5.1252954e-07}, {"x"=-5.959748, "y"=0.2976503, "Z"=5.210177e-07}, {"x"=-5.9758472, "y"=0.33151048, "Z"=5.224252e-07}, {"x"=-5.952808, "y"=0.367589, "Z"=5.20411e-07}, {"x"=-5.9215603, "y"=0.40376043, "Z"=5.1767927e-07}, {"x"=-5.947047, "y"=0.4372328, "Z"=5.1990736e-07}, {"x"=-5.9403634, "y"=0.47211158, "Z"=5.1932307e-07}, {"x"=-5.9364743, "y"=0.50681686, "Z"=5.189831e-07}, {"x"=-5.9393806, "y"=0.5413065, "Z"=5.192371e-07}, {"x"=-5.9390874, "y"=0.5758766, "Z"=5.192115e-07}, {"x"=-5.930593, "y"=0.61053234, "Z"=5.184689e-07}, {"x"=-5.921897, "y"=0.64508575, "Z"=5.1770866e-07}, {"x"=-5.8849998, "y"=0.6795378, "Z"=5.14483e-07}, {"x"=-5.8789034, "y"=0.7137373, "Z"=5.1395006e-07}, {"x"=-5.881607, "y"=0.74796987, "Z"=5.141864e-07}, {"x"=-5.901109, "y"=0.7825303, "Z"=5.158914e-07}, {"x"=-5.934404, "y"=0.81764466, "Z"=5.1880204e-07}, {"x"=-5.96449, "y"=0.85306275, "Z"=5.214323e-07}, {"x"=-6.003358, "y"=0.88914883, "Z"=5.248302e-07}, {"x"=-6.011032, "y"=0.9244334, "Z"=5.255011e-07}, {"x"=-5.98953, "y"=0.9584675, "Z"=5.2362134e-07}, {"x"=-5.948862, "y"=0.99126697, "Z"=5.2006607e-07}, {"x"=-5.946951, "y"=1.0258671, "Z"=5.1989895e-07}, {"x"=-5.9398484, "y"=1.0601362, "Z"=5.1927805e-07}, {"x"=-5.9375367, "y"=1.0946827, "Z"=5.1907597e-07}, {"x"=-5.9370184, "y"=1.1293662, "Z"=5.190306e-07}, {"x"=-5.924337, "y"=1.1630824, "Z"=5.17922e-07}, {"x"=-5.919434, "y"=1.1973629, "Z"=5.174934e-07}, {"x"=-5.8755016, "y"=1.227981, "Z"=5.1365265e-07}, {"x"=-5.8821654, "y"=1.2631369, "Z"=5.1423524e-07}, {"x"=-5.8836465, "y"=1.2978667, "Z"=5.1436473e-07}, {"x"=-5.877965, "y"=1.3318619, "Z"=5.1386803e-07}, {"x"=-5.872087, "y"=1.3658118, "Z"=5.1335417e-07}, {"x"=-5.8967824, "y"=1.4034905, "Z"=5.155131e-07}, {"x"=-5.9073515, "y"=1.4396942, "Z"=5.1643707e-07}, {"x"=-5.930582, "y"=1.4777781, "Z"=5.1846797e-07}, {"x"=-5.932773, "y"=1.5132372, "Z"=5.186595e-07}, {"x"=-5.9208994, "y"=1.5467211, "Z"=5.1762146e-07}, {"x"=-5.90686, "y"=1.5797939, "Z"=5.163941e-07}, {"x"=-5.9114027, "y"=1.6157031, "Z"=5.1679126e-07}, {"x"=-5.921648, "y"=1.6526682, "Z"=5.176869e-07}, {"x"=-5.952365, "y"=1.6933084, "Z"=5.203723e-07}, {"x"=-5.9562182, "y"=1.7296524, "Z"=5.2070914e-07}, {"x"=-5.960833, "y"=1.7662549, "Z"=5.2111255e-07}, {"x"=-5.955396, "y"=1.8010967, "Z"=5.206373e-07}, {"x"=-5.9360123, "y"=1.8332419, "Z"=5.1894267e-07}, {"x"=-5.9546967, "y"=1.87286, "Z"=5.205761e-07}, {"x"=-5.9525537, "y"=1.9084897, "Z"=5.2038877e-07}, {"x"=-5.962914, "y"=1.9468365, "Z"=5.212945e-07}, {"x"=-5.9730287, "y"=1.9853451, "Z"=5.2217877e-07}, {"x"=-5.9907017, "y"=2.0257678, "Z"=5.2372377e-07}, {"x"=-6.012978, "y"=2.0675642, "Z"=5.256712e-07}, {"x"=-6.018428, "y"=2.1057465, "Z"=5.261477e-07}, {"x"=-5.995456, "y"=2.1371899, "Z"=5.241394e-07}, {"x"=-5.9985223, "y"=2.1749434, "Z"=5.244075e-07}, {"x"=-5.949031, "y"=2.199419, "Z"=5.200808e-07}, {"x"=-5.8984914, "y"=2.2231166, "Z"=5.156625e-07}, {"x"=-5.8836193, "y"=2.2558508, "Z"=5.1436234e-07}, {"x"=-5.9023213, "y"=2.2977157, "Z"=5.159973e-07}, {"x"=-5.9255486, "y"=2.3412008, "Z"=5.180279e-07}, {"x"=-5.926359, "y"=2.3786733, "Z"=5.180988e-07}, {"x"=-5.9173374, "y"=2.4134002, "Z"=5.1731007e-07}, {"x"=-5.9282303, "y"=2.4541004, "Z"=5.1826237e-07}, {"x"=-5.9598885, "y"=2.5014155, "Z"=5.2103e-07}, {"x"=-5.97974, "y"=2.5455847, "Z"=5.227655e-07}, {"x"=-5.9897494, "y"=2.5870125, "Z"=5.2364055e-07}, {"x"=-5.9861636, "y"=2.6242948, "Z"=5.2332706e-07}, {"x"=-6.0307593, "y"=2.6776361, "Z"=5.272257e-07}, {"x"=-6.0275636, "y"=2.715564, "Z"=5.2694634e-07}, {"x"=-6.012784, "y"=2.7496164, "Z"=5.256543e-07}, {"x"=-6.020459, "y"=2.7915087, "Z"=5.2632527e-07}, {"x"=-6.0335007, "y"=2.8355787, "Z"=5.274654e-07}, {"x"=-6.0199194, "y"=2.8702981, "Z"=5.262781e-07}, {"x"=-6.032395, "y"=2.914659, "Z"=5.273687e-07}, {"x"=-6.0249076, "y"=2.9518294, "Z"=5.2671413e-07}, {"x"=-6.0424, "y"=2.9986615, "Z"=5.282434e-07}, {"x"=-6.0418506, "y"=3.0388634, "Z"=5.2819536e-07}, {"x"=-6.0772843, "y"=3.0935318, "Z"=5.312931e-07}, {"x"=-6.1122847, "y"=3.148692, "Z"=5.343529e-07}, {"x"=-6.07932, "y"=3.1766086, "Z"=5.31471e-07}, {"x"=-6.0849957, "y"=3.2204063, "Z"=5.319672e-07}, {"x"=-6.1096983, "y"=3.2725575, "Z"=5.341268e-07}, {"x"=-6.1174703, "y"=3.3179538, "Z"=5.3480625e-07}, {"x"=-6.0983577, "y"=3.3518903, "Z"=5.3313533e-07}, {"x"=-6.0909343, "y"=3.3909798, "Z"=5.324864e-07}, {"x"=-6.100575, "y"=3.4378998, "Z"=5.333292e-07}, {"x"=-6.1198716, "y"=3.489613, "Z"=5.3501617e-07}, {"x"=-6.1170197, "y"=3.5315034, "Z"=5.3476685e-07}, {"x"=-6.096713, "y"=3.5653276, "Z"=5.329916e-07}, {"x"=-6.0960503, "y"=3.6085389, "Z"=5.3293365e-07}, {"x"=-6.0959897, "y"=3.6522777, "Z"=5.3292837e-07}, {"x"=-6.125203, "y"=3.7107499, "Z"=5.354823e-07}, {"x"=-6.119087, "y"=3.7521627, "Z"=5.349476e-07}, {"x"=-6.0886374, "y"=3.781352, "Z"=5.322856e-07}, {"x"=-6.0811543, "y"=3.8222268, "Z"=5.316314e-07}, {"x"=-6.073401, "y"=3.8631191, "Z"=5.3095357e-07}, {"x"=-6.090102, "y"=3.9171696, "Z"=5.3241365e-07}, {"x"=-6.116061, "y"=3.9767406, "Z"=5.3468307e-07}, {"x"=-6.139777, "y"=4.0357633, "Z"=5.367564e-07}, {"x"=-6.2014976, "y"=4.1164994, "Z"=5.421521e-07}, {"x"=-6.416801, "y"=4.2847557, "Z"=5.6097457e-07}, {"x"=-6.5773406, "y"=4.4254436, "Z"=5.750094e-07}, {"x"=-6.599612, "y"=4.489136, "Z"=5.7695644e-07}, {"x"=-6.5730267, "y"=4.524938, "Z"=5.746322e-07}, {"x"=-6.536785, "y"=4.55495, "Z"=5.714639e-07}, {"x"=-6.5372787, "y"=4.6068134, "Z"=5.7150703e-07}, {"x"=-6.4963865, "y"=4.6338573, "Z"=5.6793215e-07}, {"x"=-6.481788, "y"=4.6768293, "Z"=5.666559e-07}, {"x"=-6.3888826, "y"=4.6710234, "Z"=5.585339e-07}, {"x"=-6.3376727, "y"=4.6904745, "Z"=5.5405695e-07}, {"x"=-6.31171, "y"=4.725655, "Z"=5.517872e-07}, {"x"=-6.238583, "y"=4.7301755, "Z"=5.4539424e-07}, {"x"=-6.1814947, "y"=4.744422, "Z"=5.4040345e-07}, {"x"=-6.142764, "y"=4.7703357, "Z"=5.370175e-07}, {"x"=-6.0981383, "y"=4.7920227, "Z"=5.331162e-07}, {"x"=-6.073289, "y"=4.8268633, "Z"=5.309438e-07}, {"x"=-0.0016451083, "y"=0.6811374, "Z"=1.4381994e-10}, {"x"=-6.4596453, "y"=5.2017484, "Z"=5.6472015e-07}, {"x"=-6.502582, "y"=5.288397, "Z"=5.6847375e-07}, {"x"=-6.4837894, "y"=5.331975, "Z"=5.6683086e-07}, {"x"=-6.493028, "y"=5.3960586, "Z"=5.6763855e-07}, {"x"=0.0, "y"=0.68, "Z"=0.0}, {"x"=-7.0161138, "y"=5.9017487, "Z"=6.133682e-07}, {"x"=-6.989613, "y"=5.9454827, "Z"=6.110514e-07}, {"x"=-7.0041914, "y"=6.0206146, "Z"=6.1232583e-07}, {"x"=-6.998339, "y"=6.080819, "Z"=6.1181424e-07}, {"x"=-6.9975395, "y"=6.1454444, "Z"=6.117443e-07}, {"x"=-7.0276036, "y"=6.2350473, "Z"=6.143726e-07}, {"x"=-7.1029325, "y"=6.362039, "Z"=6.209581e-07}, {"x"=-7.2088842, "y"=6.5158896, "Z"=6.3022065e-07}, {"x"=-7.1601167, "y"=6.5456853, "Z"=6.259573e-07}, {"x"=-7.1512794, "y"=6.6082983, "Z"=6.251847e-07}, {"x"=-7.1205034, "y"=6.653012, "Z"=6.2249416e-07}, {"x"=-7.086399, "y"=6.6949787, "Z"=6.1951266e-07}, {"x"=-7.048255, "y"=6.7334933, "Z"=6.16178e-07}, {"x"=-7.0808544, "y"=6.833427, "Z"=6.1902796e-07}, {"x"=-7.048694, "y"=6.877815, "Z"=6.162164e-07}, {"x"=-7.003556, "y"=6.910737, "Z"=6.122703e-07}, {"x"=-7.0861115, "y"=7.058415, "Z"=6.1948754e-07}, {"x"=-7.1871443, "y"=7.225441, "Z"=6.283201e-07}, {"x"=-7.2004256, "y"=7.3145723, "Z"=6.294812e-07}, {"x"=-7.218032, "y"=7.408851, "Z"=6.310204e-07}, {"x"=-7.145303, "y"=7.4191637, "Z"=6.246622e-07}, {"x"=-7.019162, "y"=7.377773, "Z"=6.1363465e-07}, {"x"=-6.992312, "y"=7.4302983, "Z"=6.112873e-07}, {"x"=-6.945772, "y"=7.4638724, "Z"=6.072187e-07}, {"x"=-6.8535547, "y"=7.45215, "Z"=5.991568e-07}, {"x"=-6.8373823, "y"=7.5152345, "Z"=5.9774294e-07}, {"x"=-6.828441, "y"=7.586181, "Z"=5.969613e-07}, {"x"=-6.711966, "y"=7.547832, "Z"=5.867787e-07}, {"x"=-6.6600904, "y"=7.5745335, "Z"=5.822436e-07}, {"x"=-6.76213, "y"=7.762151, "Z"=5.9116417e-07}, {"x"=-6.7496448, "y"=7.8319125, "Z"=5.9007266e-07}, {"x"=0.0, "y"=0.68, "Z"=0.0}, {"x"=0.0, "y"=0.68, "Z"=0.0}, {"x"=0.0, "y"=0.68, "Z"=0.0}, {"x"=0.0, "y"=0.68, "Z"=0.0}, {"x"=0.0, "y"=0.68, "Z"=0.0}, {"x"=0.0, "y"=0.68, "Z"=0.0}, {"x"=0.0, "y"=0.68, "Z"=0.0}, {"x"=0.0, "y"=0.68, "Z"=0.0}, {"x"=0.0, "y"=0.68, "Z"=0.0}, {"x"=0.0, "y"=0.68, "Z"=0.0}, {"x"=-6.6047463, "y"=8.642182, "Z"=5.774053e-07}, {"x"=-6.5773363, "y"=8.70367, "Z"=5.75009e-07}, {"x"=-6.549433, "y"=8.765107, "Z"=5.7256966e-07}, {"x"=0.0, "y"=0.68, "Z"=0.0}, {"x"=0.0, "y"=0.68, "Z"=0.0}, {"x"=0.0, "y"=0.68, "Z"=0.0}, {"x"=0.0, "y"=0.68, "Z"=0.0}, {"x"=0.0, "y"=0.68, "Z"=0.0}, {"x"=0.0, "y"=0.68, "Z"=0.0}, {"x"=0.0, "y"=0.68, "Z"=0.0}, {"x"=0.0, "y"=0.68, "Z"=0.0}, {"x"=0.0, "y"=0.68, "Z"=0.0}, {"x"=0.0, "y"=0.68, "Z"=0.0}, {"x"=0.0, "y"=0.68, "Z"=0.0}, {"x"=0.0, "y"=0.68, "Z"=0.0}, {"x"=0.0, "y"=0.68, "Z"=0.0}, {"x"=-6.206232, "y"=9.763209, "Z"=5.4256606e-07}, {"x"=0.0, "y"=0.68, "Z"=0.0}, {"x"=0.0, "y"=0.68, "Z"=0.0}, {"x"=0.0, "y"=0.68, "Z"=0.0}, {"x"=0.0, "y"=0.68, "Z"=0.0}, {"x"=0.0, "y"=0.68, "Z"=0.0}, {"x"=0.0, "y"=0.68, "Z"=0.0}, {"x"=0.0, "y"=0.68, "Z"=0.0}, {"x"=0.0, "y"=0.68, "Z"=0.0}, {"x"=0.0, "y"=0.68, "Z"=0.0}, {"x"=0.0, "y"=0.68, "Z"=0.0}, {"x"=0.0, "y"=0.68, "Z"=0.0}, {"x"=0.0, "y"=0.68, "Z"=0.0}, {"x"=0.0, "y"=0.68, "Z"=0.0}, {"x"=0.0, "y"=0.68, "Z"=0.0}, {"x"=0.0, "y"=0.68, "Z"=0.0}, {"x"=0.0, "y"=0.68, "Z"=0.0}, {"x"=0.0, "y"=0.68, "Z"=0.0}, {"x"=0.0, "y"=0.68, "Z"=0.0}, {"x"=0.0, "y"=0.68, "Z"=0.0}, {"x"=0.0, "y"=0.68, "Z"=0.0}, {"x"=0.0, "y"=0.68, "Z"=0.0}, {"x"=0.0, "y"=0.68, "Z"=0.0}, {"x"=0.0, "y"=0.68, "Z"=0.0}, {"x"=0.0, "y"=0.68, "Z"=0.0}, {"x"=0.0, "y"=0.68, "Z"=0.0}, {"x"=0.0, "y"=0.68, "Z"=0.0}, {"x"=0.0, "y"=0.68, "Z"=0.0}, {"x"=0.0, "y"=0.68, "Z"=0.0}, {"x"=0.0, "y"=0.68, "Z"=0.0}, {"x"=0.0, "y"=0.68, "Z"=0.0}, {"x"=0.0, "y"=0.68, "Z"=0.0}, {"x"=0.0, "y"=0.68, "Z"=0.0}, {"x"=0.0, "y"=0.68, "Z"=0.0}, {"x"=0.0, "y"=0.68, "Z"=0.0}, {"x"=0.0, "y"=0.68, "Z"=0.0}, {"x"=0.0, "y"=0.68, "Z"=0.0}, {"x"=0.0, "y"=0.68, "Z"=0.0}, {"x"=0.0, "y"=0.68, "Z"=0.0}, {"x"=0.0, "y"=0.68, "Z"=0.0}, {"x"=0.0, "y"=0.68, "Z"=0.0}, {"x"=0.0, "y"=0.68, "Z"=0.0}, {"x"=0.0, "y"=0.68, "Z"=0.0}, {"x"=0.0, "y"=0.68, "Z"=0.0}, {"x"=0.0, "y"=0.68, "Z"=0.0}, {"x"=0.0, "y"=0.68, "Z"=0.0}, {"x"=0.0, "y"=0.68, "Z"=0.0}, {"x"=0.0, "y"=0.68, "Z"=0.0}, {"x"=0.0, "y"=0.68, "Z"=0.0}, {"x"=0.0, "y"=0.68, "Z"=0.0}, {"x"=0.0, "y"=0.68, "Z"=0.0}, {"x"=0.0, "y"=0.68, "Z"=0.0}, {"x"=0.0, "y"=0.68, "Z"=0.0}, {"x"=0.0, "y"=0.68, "Z"=0.0}, {"x"=0.0, "y"=0.68, "Z"=0.0}, {"x"=0.0, "y"=0.68, "Z"=0.0}, {"x"=0.0, "y"=0.68, "Z"=0.0}, {"x"=0.0, "y"=0.68, "Z"=0.0}, {"x"=0.0, "y"=0.68, "Z"=0.0}, {"x"=0.0, "y"=0.68, "Z"=0.0}, {"x"=0.0, "y"=0.68, "Z"=0.0}, {"x"=0.0, "y"=0.68, "Z"=0.0}, {"x"=0.0, "y"=0.68, "Z"=0.0}, {"x"=0.0, "y"=0.68, "Z"=0.0}, {"x"=0.0, "y"=0.68, "Z"=0.0}, {"x"=0.0, "y"=0.68, "Z"=0.0}, {"x"=0.0, "y"=0.68, "Z"=0.0}, {"x"=0.0, "y"=0.68, "Z"=0.0}, {"x"=0.0, "y"=0.68, "Z"=0.0}, {"x"=0.0, "y"=0.68, "Z"=0.0}, {"x"=0.0, "y"=0.68, "Z"=0.0}, {"x"=0.0, "y"=0.68, "Z"=0.0}, {"x"=0.0, "y"=0.68, "Z"=0.0}, {"x"=0.0, "y"=0.68, "Z"=0.0}, {"x"=0.0, "y"=0.68, "Z"=0.0}, {"x"=0.0, "y"=0.68, "Z"=0.0}, {"x"=0.0, "y"=0.68, "Z"=0.0}, {"x"=0.0, "y"=0.68, "Z"=0.0}, {"x"=0.0, "y"=0.68, "Z"=0.0}, {"x"=0.0, "y"=0.68, "Z"=0.0}, {"x"=0.0, "y"=0.68, "Z"=0.0}, {"x"=0.0, "y"=0.68, "Z"=0.0}, {"x"=0.0, "y"=0.68, "Z"=0.0}, {"x"=0.0, "y"=0.68, "Z"=0.0}, {"x"=0.0, "y"=0.68, "Z"=0.0}, {"x"=0.0, "y"=0.68, "Z"=0.0}, {"x"=0.0, "y"=0.68, "Z"=0.0}, {"x"=0.0, "y"=0.68, "Z"=0.0}, {"x"=0.0, "y"=0.68, "Z"=0.0}, {"x"=0.0, "y"=0.68, "Z"=0.0}, {"x"=0.0, "y"=0.68, "Z"=0.0}, {"x"=0.0, "y"=0.68, "Z"=0.0}, {"x"=0.0, "y"=0.68, "Z"=0.0}, {"x"=0.0, "y"=0.68, "Z"=0.0}, {"x"=0.0, "y"=0.68, "Z"=0.0}, {"x"=0.0, "y"=0.68, "Z"=0.0}, {"x"=0.0, "y"=0.68, "Z"=0.0}, {"x"=0.0, "y"=0.68, "Z"=0.0}, {"x"=0.0, "y"=0.68, "Z"=0.0}, {"x"=0.0, "y"=0.68, "Z"=0.0}, {"x"=0.0, "y"=0.68, "Z"=0.0}, {"x"=0.0, "y"=0.68, "Z"=0.0}, {"x"=0.0, "y"=0.68, "Z"=0.0}, {"x"=0.0, "y"=0.68, "Z"=0.0}, {"x"=0.0, "y"=0.68, "Z"=0.0}, {"x"=0.0, "y"=0.68, "Z"=0.0}, {"x"=0.0, "y"=0.68, "Z"=0.0}, {"x"=0.0, "y"=0.68, "Z"=0.0}, {"x"=0.0, "y"=0.68, "Z"=0.0}, {"x"=0.0, "y"=0.68, "Z"=0.0}, {"x"=0.0, "y"=0.68, "Z"=0.0}, {"x"=0.0, "y"=0.68, "Z"=0.0}, {"x"=0.0, "y"=0.68, "Z"=0.0}, {"x"=0.0, "y"=0.68, "Z"=0.0}, {"x"=0.0, "y"=0.68, "Z"=0.0}, {"x"=0.0, "y"=0.68, "Z"=0.0}, {"x"=0.0, "y"=0.68, "Z"=0.0}, {"x"=0.0, "y"=0.68, "Z"=0.0}, {"x"=0.0, "y"=0.68, "Z"=0.0}, {"x"=0.0, "y"=0.68, "Z"=0.0}, {"x"=0.0, "y"=0.68, "Z"=0.0}, {"x"=0.0, "y"=0.68, "Z"=0.0}, {"x"=0.0, "y"=0.68, "Z"=0.0}, {"x"=0.0, "y"=0.68, "Z"=0.0}, {"x"=0.0, "y"=0.68, "Z"=0.0}, {"x"=0.0, "y"=0.68, "Z"=0.0}, {"x"=0.0, "y"=0.68, "Z"=0.0}, {"x"=0.0, "y"=0.68, "Z"=0.0}, {"x"=0.0, "y"=0.68, "Z"=0.0}, {"x"=0.0, "y"=0.68, "Z"=0.0}, {"x"=0.0, "y"=0.68, "Z"=0.0}, {"x"=0.0, "y"=0.68, "Z"=0.0}, {"x"=0.0, "y"=0.68, "Z"=0.0}, {"x"=0.0, "y"=0.68, "Z"=0.0}, {"x"=0.0, "y"=0.68, "Z"=0.0}, {"x"=0.0, "y"=0.68, "Z"=0.0}, {"x"=0.0, "y"=0.68, "Z"=0.0}, {"x"=0.0, "y"=0.68, "Z"=0.0}, {"x"=0.0, "y"=0.68, "Z"=0.0}, {"x"=0.0, "y"=0.68, "Z"=0.0}, {"x"=0.0, "y"=0.68, "Z"=0.0}, {"x"=0.0, "y"=0.68, "Z"=0.0}, {"x"=0.0, "y"=0.68, "Z"=0.0}, {"x"=0.0, "y"=0.68, "Z"=0.0}, {"x"=0.0, "y"=0.68, "Z"=0.0}, {"x"=0.0, "y"=0.68, "Z"=0.0}, {"x"=0.0, "y"=0.68, "Z"=0.0}, {"x"=0.0, "y"=0.68, "Z"=0.0}, {"x"=0.0, "y"=0.68, "Z"=0.0}, {"x"=0.0, "y"=0.68, "Z"=0.0}, {"x"=0.0, "y"=0.68, "Z"=0.0}, {"x"=0.0, "y"=0.68, "Z"=0.0}, {"x"=0.0, "y"=0.68, "Z"=0.0}, {"x"=0.0, "y"=0.68, "Z"=0.0}, {"x"=0.0, "y"=0.68, "Z"=0.0}, {"x"=0.0, "y"=0.68, "Z"=0.0}, {"x"=0.0, "y"=0.68, "Z"=0.0}, {"x"=0.0, "y"=0.68, "Z"=0.0}, {"x"=0.0, "y"=0.68, "Z"=0.0}, {"x"=0.0, "y"=0.68, "Z"=0.0}, {"x"=0.0, "y"=0.68, "Z"=0.0}, {"x"=0.0, "y"=0.68, "Z"=0.0}, {"x"=0.0, "y"=0.68, "Z"=0.0}, {"x"=0.0, "y"=0.68, "Z"=0.0}, {"x"=0.0, "y"=0.68, "Z"=0.0}, {"x"=0.0, "y"=0.68, "Z"=0.0}, {"x"=0.0, "y"=0.68, "Z"=0.0}, {"x"=0.0, "y"=0.68, "Z"=0.0}, {"x"=0.0, "y"=0.68, "Z"=0.0}, {"x"=0.0, "y"=0.68, "Z"=0.0}, {"x"=0.0, "y"=0.68, "Z"=0.0}, {"x"=0.0, "y"=0.68, "Z"=0.0}, {"x"=0.0, "y"=0.68, "Z"=0.0}, {"x"=0.0, "y"=0.68, "Z"=0.0}, {"x"=0.0, "y"=0.68, "Z"=0.0}, {"x"=0.0, "y"=0.68, "Z"=0.0}, {"x"=0.0, "y"=0.68, "Z"=0.0}, {"x"=0.0, "y"=0.68, "Z"=0.0}, {"x"=0.0, "y"=0.68, "Z"=0.0}, {"x"=0.0, "y"=0.68, "Z"=0.0}, {"x"=0.0, "y"=0.68, "Z"=0.0}, {"x"=0.0, "y"=0.68, "Z"=0.0}, {"x"=0.0, "y"=0.68, "Z"=0.0}, {"x"=0.0, "y"=0.68, "Z"=0.0}, {"x"=0.0, "y"=0.68, "Z"=0.0}, {"x"=0.0, "y"=0.68, "Z"=0.0}, {"x"=0.0, "y"=0.68, "Z"=0.0}, {"x"=0.0, "y"=0.68, "Z"=0.0}, {"x"=0.0, "y"=0.68, "Z"=0.0}, {"x"=0.0, "y"=0.68, "Z"=0.0}, {"x"=0.0, "y"=0.68, "Z"=0.0}, {"x"=0.0, "y"=0.68, "Z"=0.0}, {"x"=0.0, "y"=0.68, "Z"=0.0}, {"x"=0.0, "y"=0.68, "Z"=0.0}, {"x"=0.0, "y"=0.68, "Z"=0.0}, {"x"=0.0, "y"=0.68, "Z"=0.0}, {"x"=0.0, "y"=0.68, "Z"=0.0}, {"x"=0.0, "y"=0.68, "Z"=0.0}, {"x"=5.316029, "y"=9.30421, "Z"=-4.6474202e-07}, {"x"=5.351277, "y"=9.249391, "Z"=-4.6782347e-07}, {"x"=5.3833942, "y"=9.1902275, "Z"=-4.7063128e-07}, {"x"=0.0, "y"=0.68, "Z"=0.0}, {"x"=0.0, "y"=0.68, "Z"=0.0}, {"x"=0.0, "y"=0.68, "Z"=0.0}, {"x"=5.9229383, "y"=9.5779505, "Z"=-5.177997e-07}, {"x"=6.0003104, "y"=9.581489, "Z"=-5.245638e-07}, {"x"=6.0999103, "y"=9.616638, "Z"=-5.332711e-07}, {"x"=6.13701, "y"=9.559614, "Z"=-5.3651445e-07}, {"x"=6.04924, "y"=9.324669, "Z"=-5.288414e-07}, {"x"=5.994213, "y"=9.140826, "Z"=-5.240307e-07}, {"x"=6.1913676, "y"=9.312213, "Z"=-5.4126656e-07}, {"x"=6.417741, "y"=9.518808, "Z"=-5.610567e-07}, {"x"=6.4666796, "y"=9.478103, "Z"=-5.653351e-07}, {"x"=0.0, "y"=0.68, "Z"=0.0}, {"x"=5.907469, "y"=8.524375, "Z"=-5.164473e-07}, {"x"=5.778412, "y"=8.26083, "Z"=-5.051648e-07}, {"x"=5.659322, "y"=8.015687, "Z"=-4.9475364e-07}, {"x"=5.704976, "y"=7.9865823, "Z"=-4.9874484e-07}, {"x"=5.8186827, "y"=8.043502, "Z"=-5.086854e-07}, {"x"=5.830191, "y"=7.9704795, "Z"=-5.096915e-07}, {"x"=5.8221755, "y"=7.874254, "Z"=-5.0899075e-07}, {"x"=5.875332, "y"=7.85419, "Z"=-5.136378e-07}, {"x"=5.902928, "y"=7.802952, "Z"=-5.1605036e-07}, {"x"=6.019442, "y"=7.858143, "Z"=-5.2623636e-07}, {"x"=6.089565, "y"=7.856555, "Z"=-5.3236664e-07}, {"x"=6.180717, "y"=7.878672, "Z"=-5.4033546e-07}, {"x"=6.277578, "y"=7.9060087, "Z"=-5.488033e-07}, {"x"=6.357798, "y"=7.9129314, "Z"=-5.5581637e-07}, {"x"=6.4901466, "y"=7.977448, "Z"=-5.673866e-07}, {"x"=6.529143, "y"=7.935854, "Z"=-5.707958e-07}, {"x"=6.6789546, "y"=8.016062, "Z"=-5.8389276e-07}, {"x"=6.8692126, "y"=8.137428, "Z"=-6.0052565e-07}, {"x"=7.0672393, "y"=8.263409, "Z"=-6.1783766e-07}, {"x"=7.177091, "y"=8.292017, "Z"=-6.2744124e-07}, {"x"=0.0, "y"=0.68, "Z"=0.0}, {"x"=7.342941, "y"=8.288593, "Z"=-6.419403e-07}, {"x"=7.3556395, "y"=8.213552, "Z"=-6.4305044e-07}, {"x"=7.387392, "y"=8.158542, "Z"=-6.4582633e-07}, {"x"=7.4032025, "y"=8.087855, "Z"=-6.4720854e-07}, {"x"=7.436927, "y"=8.035523, "Z"=-6.501568e-07}, {"x"=0.0, "y"=0.68, "Z"=0.0}, {"x"=0.0, "y"=0.68, "Z"=0.0}, {"x"=0.0, "y"=0.68, "Z"=0.0}, {"x"=0.0, "y"=0.68, "Z"=0.0}, {"x"=6.662852, "y"=6.8971677, "Z"=-5.8248503e-07}, {"x"=6.7562423, "y"=6.911185, "Z"=-5.9064945e-07}, {"x"=0.0014780493, "y"=0.68134737, "Z"=-1.2921518e-10}, {"x"=6.9263463, "y"=6.920517, "Z"=-6.055204e-07}, {"x"=7.0080867, "y"=6.920687, "Z"=-6.126664e-07}, {"x"=5.7576256, "y"=5.74741, "Z"=-5.033476e-07}, {"x"=5.7296643, "y"=5.6639524, "Z"=-5.009032e-07}, {"x"=6.963505, "y"=6.666409, "Z"=-6.087689e-07}, {"x"=6.947913, "y"=6.583066, "Z"=-6.0740587e-07}, {"x"=6.831265, "y"=6.415871, "Z"=-5.9720816e-07}, {"x"=6.7529287, "y"=6.2834435, "Z"=-5.903598e-07}, {"x"=6.694938, "y"=6.169878, "Z"=-5.852901e-07}, {"x"=6.7267604, "y"=6.13084, "Z"=-5.8807206e-07}, {"x"=6.7380595, "y"=6.075366, "Z"=-5.890599e-07}, {"x"=6.7583523, "y"=6.0273914, "Z"=-5.908339e-07}, {"x"=6.7743764, "y"=5.976284, "Z"=-5.922348e-07}, {"x"=6.805071, "y"=5.936787, "Z"=-5.9491816e-07}, {"x"=6.807713, "y"=5.875877, "Z"=-5.951492e-07}, {"x"=6.834629, "y"=5.8337793, "Z"=-5.9750226e-07}, {"x"=6.8364263, "y"=5.773024, "Z"=-5.976594e-07}, {"x"=6.8280845, "y"=5.7053103, "Z"=-5.969301e-07}, {"x"=6.8183784, "y"=5.637279, "Z"=-5.960816e-07}, {"x"=6.824358, "y"=5.581198, "Z"=-5.966043e-07}, {"x"=6.8486753, "y"=5.5385237, "Z"=-5.987302e-07}, {"x"=6.840788, "y"=5.4733524, "Z"=-5.980407e-07}, {"x"=6.846354, "y"=5.4181128, "Z"=-5.9852727e-07}, {"x"=6.83087, "y"=5.3488636, "Z"=-5.9717365e-07}, {"x"=6.8380218, "y"=5.295621, "Z"=-5.977989e-07}, {"x"=6.8081737, "y"=5.2180495, "Z"=-5.951894e-07}, {"x"=6.834457, "y"=5.178369, "Z"=-5.974872e-07}, {"x"=5.3789005, "y"=4.175662, "Z"=-4.7023843e-07}, {"x"=5.3940945, "y"=4.1410728, "Z"=-4.7156672e-07}, {"x"=5.5298705, "y"=4.1829486, "Z"=-4.834366e-07}, {"x"=6.9839015, "y"=5.0472975, "Z"=-6.1055204e-07}, {"x"=6.9955735, "y"=4.9981933, "Z"=-6.115725e-07}, {"x"=7.009473, "y"=4.9506617, "Z"=-6.127876e-07}, {"x"=5.7307115, "y"=4.126, "Z"=-5.009947e-07}, {"x"=5.9260955, "y"=4.1967134, "Z"=-5.180757e-07}, {"x"=0.0, "y"=0.68, "Z"=0.0}, {"x"=6.677475, "y"=4.538273, "Z"=-5.837634e-07}, {"x"=6.6329126, "y"=4.4612293, "Z"=-5.798676e-07}, {"x"=6.657411, "y"=4.4240513, "Z"=-5.8200936e-07}, {"x"=6.6204896, "y"=4.3527584, "Z"=-5.7878157e-07}, {"x"=6.6075296, "y"=4.2954636, "Z"=-5.7764856e-07}, {"x"=6.6134887, "y"=4.248892, "Z"=-5.7816953e-07}, {"x"=6.591764, "y"=4.187811, "Z"=-5.762703e-07}, {"x"=6.5704393, "y"=4.1275682, "Z"=-5.7440604e-07}, {"x"=6.549526, "y"=4.068153, "Z"=-5.725778e-07}, {"x"=6.5477443, "y"=4.019093, "Z"=-5.72422e-07}, {"x"=6.53936, "y"=3.967025, "Z"=-5.71689e-07}, {"x"=6.5494094, "y"=3.92449, "Z"=-5.7256756e-07}, {"x"=6.5501995, "y"=3.8775625, "Z"=-5.726366e-07}, {"x"=6.565085, "y"=3.8376713, "Z"=-5.7393794e-07}, {"x"=6.5896683, "y"=3.8024251, "Z"=-5.760871e-07}, {"x"=6.591409, "y"=3.7564263, "Z"=-5.762393e-07}, {"x"=6.62464, "y"=3.7251313, "Z"=-5.791444e-07}, {"x"=6.638598, "y"=3.6848936, "Z"=-5.8036466e-07}, {"x"=6.6258235, "y"=3.6327922, "Z"=-5.792479e-07}, {"x"=6.641972, "y"=3.5937972, "Z"=-5.806596e-07}, {"x"=6.623005, "y"=3.539651, "Z"=-5.790015e-07}, {"x"=6.653333, "y"=3.5069413, "Z"=-5.8165284e-07}, {"x"=6.695499, "y"=3.4789894, "Z"=-5.853391e-07}, {"x"=6.711668, "y"=3.4399934, "Z"=-5.8675266e-07}, {"x"=6.7081413, "y"=3.3930302, "Z"=-5.8644434e-07}, {"x"=6.731244, "y"=3.3569183, "Z"=-5.8846405e-07}, {"x"=6.760672, "y"=3.3231783, "Z"=-5.910367e-07}, {"x"=6.7778006, "y"=3.2845232, "Z"=-5.9253415e-07}, {"x"=6.7741265, "y"=3.2379863, "Z"=-5.922129e-07}, {"x"=6.7776413, "y"=3.194363, "Z"=-5.925202e-07}, {"x"=6.7780595, "y"=3.1497586, "Z"=-5.925568e-07}, {"x"=6.8214993, "y"=3.1207314, "Z"=-5.963544e-07}, {"x"=6.8157687, "y"=3.074049, "Z"=-5.958534e-07}, {"x"=6.8295803, "y"=3.0343602, "Z"=-5.970609e-07}, {"x"=6.8545275, "y"=2.9984365, "Z"=-5.9924184e-07}, {"x"=6.8821354, "y"=2.9632466, "Z"=-6.0165536e-07}, {"x"=6.8658214, "y"=2.9135835, "Z"=-6.0022916e-07}, {"x"=6.869171, "y"=2.8705678, "Z"=-6.00522e-07}, {"x"=6.8951607, "y"=2.8347478, "Z"=-6.027941e-07}, {"x"=6.913316, "y"=2.7963574, "Z"=-6.043813e-07}, {"x"=6.890068, "y"=2.7454813, "Z"=-6.023489e-07}, {"x"=6.8664637, "y"=2.6949475, "Z"=-6.002853e-07}, {"x"=6.8723016, "y"=2.653314, "Z"=-6.0079566e-07}, {"x"=6.8682604, "y"=2.6089773, "Z"=-6.004424e-07}, {"x"=6.8909373, "y"=2.5721684, "Z"=-6.0242485e-07}, {"x"=6.876716, "y"=2.5253122, "Z"=-6.011816e-07}, {"x"=6.8844323, "y"=2.4845173, "Z"=-6.018562e-07}, {"x"=6.893844, "y"=2.4441912, "Z"=-6.02679e-07}, {"x"=6.901079, "y"=2.403332, "Z"=-6.033115e-07}, {"x"=6.873095, "y"=2.3539295, "Z"=-6.0086506e-07}, {"x"=6.822393, "y"=2.299599, "Z"=-5.964325e-07}, {"x"=6.825853, "y"=2.2585328, "Z"=-5.96735e-07}, {"x"=6.577367, "y"=2.160814, "Z"=-5.7501165e-07}, {"x"=6.1912255, "y"=2.036087, "Z"=-5.412541e-07}, {"x"=6.140325, "y"=1.9875524, "Z"=-5.368043e-07}, {"x"=6.061652, "y"=1.9339838, "Z"=-5.2992647e-07}, {"x"=5.9855075, "y"=1.8819661, "Z"=-5.232697e-07}, {"x"=5.9629517, "y"=1.8413918, "Z"=-5.212978e-07}, {"x"=5.924405, "y"=1.7981536, "Z"=-5.1792796e-07}, {"x"=5.900314, "y"=1.7580996, "Z"=-5.158218e-07}, {"x"=5.8651266, "y"=1.7164495, "Z"=-5.1274566e-07}, {"x"=5.8631706, "y"=1.6809673, "Z"=-5.125747e-07}, {"x"=5.856067, "y"=1.6447303, "Z"=-5.1195366e-07}, {"x"=5.8161488, "y"=1.6034353, "Z"=-5.0846387e-07}, {"x"=5.7838583, "y"=1.563846, "Z"=-5.0564097e-07}, {"x"=5.7651567, "y"=1.5266981, "Z"=-5.04006e-07}, {"x"=5.746219, "y"=1.4897978, "Z"=-5.023504e-07}, {"x"=5.7438955, "y"=1.455421, "Z"=-5.021473e-07}, {"x"=5.739383, "y"=1.4208426, "Z"=-5.017528e-07}, {"x"=5.7326784, "y"=1.3860986, "Z"=-5.0116665e-07}, {"x"=5.721791, "y"=1.3509917, "Z"=-5.002148e-07}, {"x"=5.727585, "y"=1.3179172, "Z"=-5.0072134e-07}, {"x"=5.7302046, "y"=1.2844833, "Z"=-5.009504e-07}, {"x"=5.722678, "y"=1.2500494, "Z"=-5.002924e-07}, {"x"=5.7249017, "y"=1.2166567, "Z"=-5.004868e-07}, {"x"=5.7249384, "y"=1.1830823, "Z"=-5.0049e-07}, {"x"=5.718798, "y"=1.1490353, "Z"=-4.999532e-07}, {"x"=5.715447, "y"=1.1153046, "Z"=-4.9966025e-07}, {"x"=5.703917, "y"=1.0810677, "Z"=-4.9865224e-07}, {"x"=5.697172, "y"=1.0473013, "Z"=-4.980626e-07}, {"x"=5.698214, "y"=1.0140953, "Z"=-4.9815367e-07}, {"x"=5.685082, "y"=0.9801514, "Z"=-4.9700566e-07}, {"x"=5.6837354, "y"=0.9469346, "Z"=-4.9688794e-07}, {"x"=5.691187, "y"=0.9141135, "Z"=-4.9753936e-07}, {"x"=5.7054443, "y"=0.88146186, "Z"=-4.9878577e-07}, {"x"=5.7245116, "y"=0.8487996, "Z"=-5.004527e-07}, {"x"=5.7303953, "y"=0.81561464, "Z"=-5.009671e-07}, {"x"=5.738086, "y"=0.7824027, "Z"=-5.016394e-07}, {"x"=5.7465844, "y"=0.74911785, "Z"=-5.0238236e-07}, {"x"=5.7328897, "y"=0.715601, "Z"=-5.011851e-07}, {"x"=5.7479997, "y"=0.68225724, "Z"=-5.025061e-07}, {"x"=5.7589154, "y"=0.64876056, "Z"=-5.034604e-07}, {"x"=5.7626357, "y"=0.61521566, "Z"=-5.037856e-07}, {"x"=5.7891574, "y"=0.5812341, "Z"=-5.061042e-07}, {"x"=5.7914844, "y"=0.5474907, "Z"=-5.0630763e-07}, {"x"=5.8036103, "y"=0.51343006, "Z"=-5.073677e-07}, {"x"=5.827528, "y"=0.47880983, "Z"=-5.094587e-07}, {"x"=5.83725, "y"=0.44447017, "Z"=-5.103086e-07}, {"x"=5.8627524, "y"=0.40927252, "Z"=-5.125381e-07}, {"x"=5.886045, "y"=0.37387413, "Z"=-5.1457437e-07}, {"x"=5.8841643, "y"=0.3396393, "Z"=-5.1441e-07}, {"x"=5.886077, "y"=0.30516177, "Z"=-5.145772e-07}, {"x"=5.9017534, "y"=0.2696795, "Z"=-5.1594765e-07}, {"x"=5.9521165, "y"=0.23137158, "Z"=-5.2035057e-07}, {"x"=5.9832945, "y"=0.19400221, "Z"=-5.230762e-07}, {"x"=6.0112495, "y"=0.1565153, "Z"=-5.2552014e-07}, {"x"=6.0728235, "y"=0.11554009, "Z"=-5.309031e-07}, {"x"=6.1450686, "y"=0.07274926, "Z"=-5.3721897e-07}, {"x"=6.2926064, "y"=0.021185338, "Z"=-5.5011714e-07}, {"x"=6.47851, "y"=-0.03640157, "Z"=-5.6636935e-07}, {"x"=6.6977224, "y"=-0.10010648, "Z"=-5.855335e-07}, {"x"=6.8042417, "y"=-0.15265924, "Z"=-5.948457e-07}, {"x"=6.8369737, "y"=-0.19706154, "Z"=-5.9770724e-07}, {"x"=6.8377028, "y"=-0.23761648, "Z"=-5.9777096e-07}, {"x"=6.857998, "y"=-0.28098494, "Z"=-5.995452e-07}, {"x"=6.873071, "y"=-0.32389778, "Z"=-6.0086296e-07}, {"x"=6.8928194, "y"=-0.36776978, "Z"=-6.025894e-07}, {"x"=6.914265, "y"=-0.41221756, "Z"=-6.044643e-07}, {"x"=6.9176626, "y"=-0.45403808, "Z"=-6.047613e-07}, {"x"=6.9306664, "y"=-0.49761027, "Z"=-6.058981e-07}, {"x"=6.937487, "y"=-0.5403324, "Z"=-6.064944e-07}, {"x"=6.2287827, "y"=-0.45306224, "Z"=-5.445375e-07}, {"x"=6.1572213, "y"=-0.4770872, "Z"=-5.3828137e-07}, {"x"=6.1513677, "y"=-0.51307553, "Z"=-5.3776967e-07}, {"x"=6.1580515, "y"=-0.5515843, "Z"=-5.3835396e-07}, {"x"=8.640479, "y"=-1.1003945, "Z"=-7.553747e-07}, {"x"=6.966001, "y"=-0.7976578, "Z"=-6.0898714e-07}, {"x"=6.9729195, "y"=-0.84156615, "Z"=-6.09592e-07}, {"x"=6.9776106, "y"=-0.8851672, "Z"=-6.100021e-07}, {"x"=6.977158, "y"=-0.9277515, "Z"=-6.099625e-07}, {"x"=6.9822845, "y"=-0.9717646, "Z"=-6.104107e-07}, {"x"=6.9745016, "y"=-1.0128253, "Z"=-6.097303e-07}, {"x"=6.957743, "y"=-1.051678, "Z"=-6.082652e-07}, {"x"=6.958211, "y"=-1.0948415, "Z"=-6.083061e-07}, {"x"=6.9758267, "y"=-1.1426194, "Z"=-6.0984615e-07}, {"x"=6.9815288, "y"=-1.187561, "Z"=-6.103446e-07}, {"x"=6.9618664, "y"=-1.2257657, "Z"=-6.0862567e-07}, {"x"=6.9660697, "y"=-1.270546, "Z"=-6.0899316e-07}, {"x"=6.9478755, "y"=-1.309109, "Z"=-6.0740257e-07}, {"x"=6.9323483, "y"=-1.3483686, "Z"=-6.0604515e-07}, {"x"=6.935761, "y"=-1.3932433, "Z"=-6.0634346e-07}, {"x"=6.941756, "y"=-1.4391019, "Z"=-6.0686756e-07}, {"x"=6.918809, "y"=-1.4761746, "Z"=-6.048615e-07}, {"x"=6.8680305, "y"=-1.5042629, "Z"=-6.004223e-07}, {"x"=6.8761344, "y"=-1.5509677, "Z"=-6.0113075e-07}, {"x"=6.8744326, "y"=-1.5946991, "Z"=-6.00982e-07}, {"x"=6.871507, "y"=-1.6381664, "Z"=-6.0072625e-07}, {"x"=6.815351, "y"=-1.6634674, "Z"=-5.958169e-07}, {"x"=6.59681, "y"=-1.6313202, "Z"=-5.7671144e-07}, {"x"=6.3835893, "y"=-1.598393, "Z"=-5.580711e-07}, {"x"=6.7010508, "y"=-1.7557383, "Z"=-5.8582447e-07}, {"x"=6.847138, "y"=-1.8540287, "Z"=-5.985958e-07}, {"x"=6.8350887, "y"=-1.8948743, "Z"=-5.9754245e-07}, {"x"=6.8199944, "y"=-1.9345915, "Z"=-5.9622283e-07}, {"x"=6.8829274, "y"=-2.0047452, "Z"=-6.0172465e-07}, {"x"=5.8047676, "y"=-1.6231935, "Z"=-5.074689e-07}, {"x"=5.58911, "y"=-1.5753446, "Z"=-4.886155e-07}, {"x"=6.824852, "y"=-2.1202724, "Z"=-5.966475e-07}, {"x"=6.8259826, "y"=-2.1672406, "Z"=-5.9674636e-07}, {"x"=6.821273, "y"=-2.2119746, "Z"=-5.963346e-07}, {"x"=6.813518, "y"=-2.2555628, "Z"=-5.956567e-07}, {"x"=6.7981586, "y"=-2.2959504, "Z"=-5.943139e-07}, {"x"=6.801748, "y"=-2.344792, "Z"=-5.946277e-07}, {"x"=6.8332496, "y"=-2.4065363, "Z"=-5.9738164e-07}, {"x"=6.8069983, "y"=-2.4424818, "Z"=-5.950867e-07}, {"x"=6.766057, "y"=-2.4714706, "Z"=-5.915075e-07}, {"x"=6.8108916, "y"=-2.5407007, "Z"=-5.954271e-07}, {"x"=6.7514725, "y"=-2.560793, "Z"=-5.9023245e-07}, {"x"=6.8206067, "y"=-2.642934, "Z"=-5.962764e-07}, {"x"=0.0, "y"=0.68, "Z"=0.0}, {"x"=0.0017876594, "y"=0.6791032, "Z"=-1.5628214e-10}, {"x"=7.081524, "y"=-2.9242942, "Z"=-6.190865e-07}, {"x"=6.786763, "y"=-2.8241248, "Z"=-5.933177e-07}, {"x"=6.6900797, "y"=-2.8236465, "Z"=-5.8486535e-07}, {"x"=6.6157126, "y"=-2.8338904, "Z"=-5.78364e-07}, {"x"=6.5872364, "y"=-2.8680477, "Z"=-5.758745e-07}, {"x"=6.605101, "y"=-2.9273968, "Z"=-5.7743625e-07}, {"x"=6.61025, "y"=-2.9802914, "Z"=-5.778864e-07}, {"x"=6.6228538, "y"=-3.037773, "Z"=-5.7898825e-07}, {"x"=6.6706457, "y"=-3.1158013, "Z"=-5.8316635e-07}, {"x"=6.5990763, "y"=-3.1260633, "Z"=-5.7690954e-07}, {"x"=6.5017147, "y"=-3.1204827, "Z"=-5.68398e-07}, {"x"=6.4657307, "y"=-3.1500852, "Z"=-5.6525215e-07}, {"x"=5.001199, "y"=-2.3219829, "Z"=-4.372187e-07}, {"x"=4.954602, "y"=-2.333357, "Z"=-4.3314503e-07}, {"x"=4.9574213, "y"=-2.3747182, "Z"=-4.3339153e-07}, {"x"=0.0016965714, "y"=0.67894095, "Z"=-1.4831898e-10}, {"x"=0.31525624, "y"=0.48064476, "Z"=-2.7560576e-08}, {"x"=0.31324914, "y"=0.4793536, "Z"=-2.738511e-08}, {"x"=0.30452642, "y"=0.48243314, "Z"=-2.6622544e-08}, {"x"=0.29752183, "y"=0.48450893, "Z"=-2.6010184e-08}, {"x"=0.2963796, "y"=0.48278153, "Z"=-2.5910326e-08}, {"x"=0.29771522, "y"=0.4793843, "Z"=-2.6027092e-08}, {"x"=0.29571712, "y"=0.4782195, "Z"=-2.5852412e-08}, {"x"=0.29207015, "y"=0.47820795, "Z"=-2.5533584e-08}, {"x"=0.2933496, "y"=0.47479272, "Z"=-2.5645436e-08}, {"x"=0.2872545, "y"=0.47655752, "Z"=-2.5112588e-08}, {"x"=0.28444082, "y"=0.47605535, "Z"=-2.4866607e-08}, {"x"=0.2735382, "y"=0.48145318, "Z"=-2.3913469e-08}, {"x"=0.2747962, "y"=0.47808897, "Z"=-2.4023446e-08}, {"x"=0.27361697, "y"=0.47649387, "Z"=-2.3920355e-08}, {"x"=0.27482525, "y"=0.4731013, "Z"=-2.4025987e-08}, {"x"=0.26884466, "y"=0.4751426, "Z"=-2.3503148e-08}, {"x"=0.26764843, "y"=0.47358215, "Z"=-2.3398568e-08}, {"x"=0.26407826, "y"=0.47387463, "Z"=-2.3086455e-08}, {"x"=0.2644441, "y"=0.47110218, "Z"=-2.3118439e-08}, {"x"=0.26088122, "y"=0.47144067, "Z"=-2.280696e-08}, {"x"=0.25499895, "y"=0.4737004, "Z"=-2.2292717e-08}, {"x"=0.24915199, "y"=0.47602135, "Z"=-2.1781558e-08}, {"x"=0.2479612, "y"=0.47457546, "Z"=-2.1677456e-08}, {"x"=0.24446298, "y"=0.4750638, "Z"=-2.1371633e-08}, {"x"=0.2432667, "y"=0.4736452, "Z"=-2.126705e-08}, {"x"=0.24054456, "y"=0.4735362, "Z"=-2.1029074e-08}, {"x"=0.2408495, "y"=0.47082895, "Z"=-2.1055731e-08}, {"x"=0.24338457, "y"=0.466131, "Z"=-2.1277355e-08}, {"x"=0.24512568, "y"=0.46206105, "Z"=-2.1429567e-08}, {"x"=0.24608412, "y"=0.4586324, "Z"=-2.1513358e-08}, {"x"=0.24035491, "y"=0.46124327, "Z"=-2.1012493e-08}, {"x"=0.24569893, "y"=0.45375228, "Z"=-2.1479682e-08}, {"x"=0.24291532, "y"=0.45369017, "Z"=-2.1236332e-08}, {"x"=0.23868394, "y"=0.4550245, "Z"=-2.0866413e-08}, {"x"=0.24171335, "y"=0.44949913, "Z"=-2.1131251e-08}, {"x"=0.2425274, "y"=0.446014, "Z"=-2.1202418e-08}, {"x"=0.23973092, "y"=0.4460041, "Z"=-2.0957943e-08}, {"x"=0.24121185, "y"=0.44180292, "Z"=-2.108741e-08}, {"x"=0.23628493, "y"=0.44393766, "Z"=-2.0656683e-08}], 3 "data out":string="\u0002sRA LMDscandata 1 1 127E169 0 0 469E 46A0 4D0BFA83 4D0C0E59 0 0 1 0 0 5DC A2 0 1 DIST1 3F800000 00000000 FFF92230 D05 32B 14E 14B 14A 14F 14D 148 146 141 13D 14B 146 146 14A 145 149 140 142 152 143 152 150 150 2 150 155 15C 157 15C 159 159 15B 164 167 175 177 16E 17A 17A 17B 180 18A 18ED 18D4 18BE 18B5 18B0 18A2 1891 188B 187E 187F 187B 186F 1861 1855 1845 184A 1841 183E 1840 184F 185B 185C 184E 184F 184E 185C 1867 1861 185A 1871 1880 188E 1893 188C 1890 1880 186F 1851 183B 181A 17F7 17F6 1819 1852 183F 1828 180A 1821 1879 18C3 1871 17C3 17D4 1784 1793 17AC 17AC 17CF 17F3 17CD 17D8 17FC 1821 1824 17E5 17A7 179F 178D 177D 179F 1795 1785 1752 170C 1718 1726 1709 16ED 16DB 16E0 16D4 16E0 16F5 1754 1762 1749 1728 1740 1738 1733 1735 1734 172B 1722 16FD 16F7 16FA 170E 1730 174F 1777 1780 176C 1745 1745 1740 1740 1742 1738 1736 170D 1717 171C 171A 1718 1735 1744 1760 1767 1760 1757 1761 1771 1796 17A0 17AB 17AC 179F 17B9 17BE 17D0 17E2 17FC 181B 1829 181A 1826 17FC 17D1 17CB 17E8 180A 1815 1816 182C 1858 1878 188E 1896 18D1 18DA 18D7 18EC 1907 1906 1921 1927 1948 1956 198B 19C0 19AC 19C2 19ED 1A06 1A02 1A0B 1A27 1A4E 1A5D 1A59 1A6B 1A7E 1AB2 1ABF 1AB1 1ABD 1AC9 1AF1 1B24 1B55 1BB2 1CC0 1D91 1DC4 1DBF 1DAF 1DCA 1DB5 1DBF 1D6D 1D4C 1D49 1D0E 1CE6 1CD4 1CBB 1CBA 2 1ECD 1F22 1F2C 1F59 0 222A 222F 2268 2288 22AF 22FE 2388 243B 2428 2449 244E 244F 244B 24A5 24AA 249E 253E 25F9 263F 268C 265E 25E6 25F7 25ED 25A3 25C4 25F0 2583 2572 2640 266A 0 0 0 0 0 0 0 0 0 0 2869 2887 28A5 0 0 0 0 0 0 0 0 0 0 0 0 0 2AF9 0 0 0 0 0 0 0 0 0 0 0 0 0 0 0 0 0 0 0 0 0 0 0 0 0 0 0 0 0 0 0 0 0 0 0 0 0 0 0 0 0 0 0 0 0 0 0 0 0 0 0 0 0 0 0 0 0 0 0 0 0 0 0 0 0 0 0 0 0 0 0 0 0 0 0 0 0 0 0 0 0 0 0 0 0 0 0 0 0 0 0 0 0 0 0 0 0 0 0 0 0 0 0 0 0 0 0 0 0 0 0 0 0 0 0 0 0 0 0 0 0 0 0 0 0 0 0 0 0 0 0 0 0 0 0 0 0 0 0 0 0 0 0 0 0 0 0 0 0 0 0 0 0 0 0 0 0 0 0 0 0 0 0 0 0 0 0 0 0 0 0 0 0 0 0 0 0 0 0 0 0 0 0 0 0 0 0 0 0 0 0 0 0 0 0 0 0 2793 2777 2756 0 0 0 29C1 29EF 2A44 2A2A 2937 2881 297F 2AAB 2AA7 0 265C 253C 2431 2436 24A9 2477 2427 2439 2423 2498 24C4 2510 2564 259E 2626 2621 26C1 279B 287E 28DE 0 294E 2921 2910 28E9 28DC 0 0 0 0 2399 23E7 2 246B 24A8 1DF6 1DAA 23DF 239D 22D8 2247 21D2 21D2 21B8 21AA 2197 2197 2174 2170 214D 211E 20EE 20D2 20CD 20A1 2086 2052 203A 1FF6 1FF6 190F 1909 1992 202D 201D 2010 1A1F 1AEB 0 1E20 1DD3 1DD6 1D93 1D6C 1D5B 1D2B 1CFC 1CCE 1CB6 1C97 1C8D 1C79 1C75 1C7C 1C6A 1C7B 1C77 1C56 1C55 1C2E 1C3D 1C59 1C59 1C44 1C4C 1C5B 1C5D 1C49 1C3D 1C2E 1C4D 1C38 1C38 1C44 1C53 1C34 1C2A 1C38 1C3E 1C19 1BF4 1BEE 1BDE 1BEA 1BD0 1BCD 1BCC 1BC9 1BA2 1B64 1B5E 1A56 18C2 1886 182E 17D9 17BB 178D 176E 1744 173C 172F 1701 16DB 16C3 16AB 16A4 169B 1690 1681 1683 1682 1677 1676 1673 166A 1664 1656 164D 164C 163D 163A 1640 164D 165F 1664 166B 1673 1665 1674 167F 1683 169E 16A1 16AE 16C7 16D2 16ED 1706 1706 170A 171C 1751 1773 1792 17D3 181F 18B7 1976 1A57 1AC7 1AED 1AF3 1B0D 1B22 1B3C 1B58 1B62 1B76 1B84 18BB 1879 187A 1888 2276 1BD1 1BE1 1BEF 1BF8 1C07 1C09 1C02 1C0D 1C2A 1C3B 1C32 1C42 1C3B 1C37 1C47 1C5A 1C4F 1C27 1C3D 1C49 1C54 1C27 1B4E 1A7A 1BDA 1C85 1C88 1C88 1CDC 1865 178B 1CD1 1CE4 1CF1 1CFB 1CFD 1D14 1D4A 1D41 1D28 1D6E 1D41 1DA3 0 2 1F0A 1DD6 1D80 1D43 1D3A 1D66 1D84 1DAB 1DFB 1DC2 1D6B 1D5B 16C9 16A7 16BF 2 175 174 16B 164 164 167 166 163 166 160 15E 152 155 155 158 152 152 14F 151 14E 148 142 142 13F 13F 13D 13F 144 148 14B 145 14E 14C 148 14E 151 14F 153 14E 0 0 1 B not defined 0 0 0\u0003")   [LabVIEW 2019]
uses:
  Ctrl/tim571-databuf.ctl
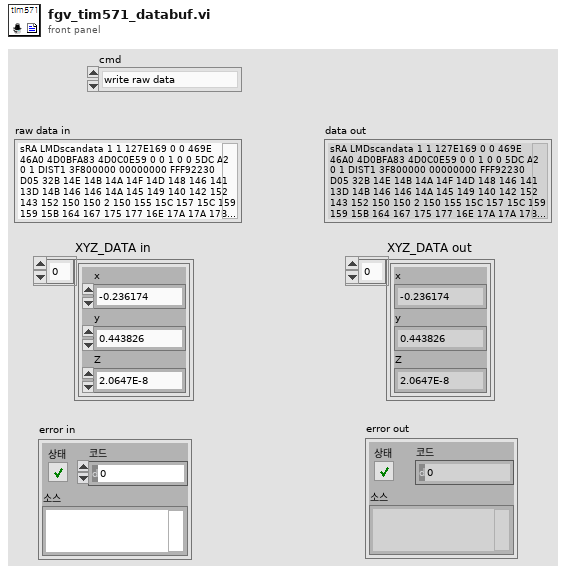
[diagram p1: front panel]
types:
  T1 = typedef "tim571-databuf.ctl" = enum16{"write raw data", "write xyz data", "read"}
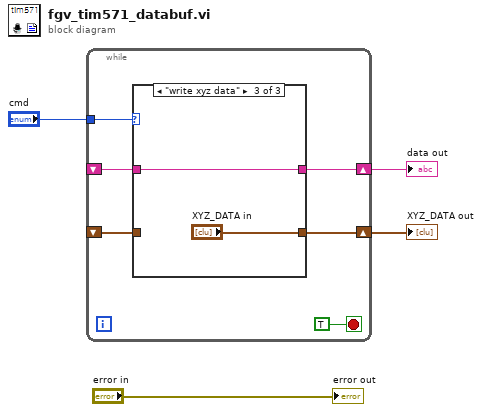
[diagram p0: block diagram]
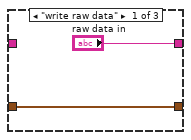
[diagram p2: hidden frame]
diagram:
  n1 = while {
    tunnel: "cmd" -> [w9]
    shift-right: [w8] -> w3
    shift-left: _ -> [w7]
    shift-right: [w6] -> w2
    shift-left: _ -> [w5]
    stop <- TRUE stop-if-true
    n2 = case shown="\"write xyz data\"" w9 {
      tunnel: ["raw data in" w14 w15] -> w8
      tunnel: w7 -> [_ w14 w15]
      tunnel: [w11 w13 "XYZ_DATA in"] -> w6
      tunnel: w5 -> [w11 w13 _]
      frame "write raw data" {
      }
      frame "read", Default {
      }
      frame "write xyz data" {
      }
    }
  }
  "data out" <- w3
  "XYZ_DATA out" <- w2
  "error out" <- "error in"
